vi "test_gpsparsing-dyy1.vi"() -> ()   [LabVIEW 2019]
panel:
  in  "rs232 input":string="INSPVAXA,USB3,0,51.0,FINESTEERING,2107,281115.600,02000000,471d,15824;INS_ALIGNMENT_COMPLETE,INS_RTKFIXED,37.37013888668,126.72084169564,9.8834,22.3000,0.0026,0.0071,0.0017,-0.044376618,-0.064379115,35.875304095,0.1980,0.1670,0.2645,0.0373,0.0373,0.0312,0.3280,0.3375,5.4270,0f000015,0*6411398e\n\t"
  in  "raw sentences":string="#INSPVAXA,USB1,0,48.5,FINESTEERING,2089,274774.000,02000000,471d,15824;INS_SOLUTION_GOOD,INS_PSRSP,37.29130387489,127.14837722879,180.1875,23.4000,-0.0013,0.0009,0.0006,0.551873578,0.409746986,245.238942969,0.9351,1.1352,1.8213,0.0013,0.0013,0.0011,0.5220,0.5327,0.0827,0f000044,0*ebcb680a\r\n#INSPVAXA,USB1,0,46.0,FINESTEERING,2089,274774.500,02000000,471d,15824;INS_SOLUTION_GOOD,INS_PSRSP,37.29130387510,127.14837722993,180.1872,23.4000,-0.0011,0.0012,0.0001,0.555094420,0.409664932,245.237706469,0.9353,1.1353,1.8214,0.0013,0.0013,0.0011,0.5219,0.5326,0.0825,0f000044,0*777011ab\r\n#INSPVAXA,USB1,0,43.5,FINESTEERING,2089,274833.000,02000000,471d,15824;INS_SOLUTION_GOOD,INS_PSRSP,37.29130384920,127.14837718901,180.1935,23.4000,0.0010,0.0016,0.0001,0.586508598,0.420271557,245.302228537,0.9484,1.1462,1.8280,0.0013,0.0013,0.0011,0.5170,0.5273,0.0804,0f000044,0*4ffbbfb3\r\n#INSPVAXA,USB1,0,43.5,FINESTEERING,2089,274833.500,02000000,471d,15824;INS_SOLUTION_GOOD,INS_PSRSP,37.29130384818,127.14837718608,180.1933,23.4000,0.0010,0.0008,-0.0005,0.588637214,0.418146390,245.299960128,0.9485,1.1462,1.8281,0.0013,0.0013,0.0011,0.5169,0.5272,0.0802,0f000044,0*aa66d913\r\n#INSPVAXA,USB1,0,45.5,FINESTEERING,2089,274834.000,02000000,471d,15824;INS_SOLUTION_GOOD,INS_PSRSP,37.29130384916,127.14837718345,180.1929,23.4000,0.0015,0.0004,-0.0005,0.590372743,0.418871037,245.299569777,0.9485,1.1462,1.8281,0.0013,0.0013,0.0011,0.5169,0.5272,0.0802,0f000044,0*83fcb3d7\r\n#INSPVAXA,USB1,0,41.5,FINESTEERING,2089,274834.500,02000000,471d,15824;INS_SOLUTION_GOOD,INS_PSRSP,37.29130384548,127.14837718346,180.1928,23.4000,0.0001,0.0000,-0.0006,0.589131920,0.420278401,245.300229975,0.9486,1.1463,1.8281,0.0013,0.0013,0.0011,0.5168,0.5272,0.0801,0f000044,0*a2231570\r\n#INSPVAXA,USB1,0,41.5,FINESTEERING,2089,274835.000,02000000,471d,15824;INS_SOLUTION_GOOD,INS_PSRSP,37.29130384335,127.14837718516,180.1928,23.4000,0.0007,0.0007,-0.0001,0.587725622,0.422163583,245.298857552,0.9486,1.1463,1.8281,0.0013,0.0013,0.0011,0.5168,0.5272,0.0801,0f000044,0*a4c2c19e\r\n#INSPVAXA,USB1,0,41.5,FINESTEERING,2089,274835.500,02000000,471d,15824;INS_SOLUTION_GOOD,INS_PSRSP,37.29130384579,127.14837718571,180.1931,23.4000,0.0007,0.0010,0.0003,0.585320450,0.422207630,245.298031526,0.9487,1.1464,1.8282,0.0013,0.0013,0.0011,0.5167,0.5271,0.0801,0f000044,0*54c9d66f\r\n#INSPVAXA,USB1,0,42.0,FINESTEERING,2089,274836.000,02000000,471d,15824;INS_SOLUTION_GOOD,INS_PSRSP,37.29130384541,127.14837718965,180.1938,23.4000,-0.0004,0.0017,0.0013,0.584834735,0.420652895,245.296961531,0.9487,1.1464,1.8282,0.0013,0.0013,0.0011,0.5167,0.5271,0.0801,0f000044,0*6e73d9be\r\n#INSPVAXA,USB1,0,42.0,FINESTEERING,2089,274836.500,02000000,471d,15824;INS_SOLUTION_GOOD,INS_PSRSP,37.29130384325,127.14837718988,180.1936,23.4000,-0.0007,0.0022,0.0002,0.586640561,0.420248412,245.293704375,0.9488,1.1465,1.8282,0.0013,0.0013,0.0011,0.5166,0.5269,0.0800,0f000044,0*6525d3dd\r\n#INSPVAXA,USB1,0,46.5,FINESTEERING,2089,274837.000,02000000,471d,15824;INS_SOLUTION_GOOD,INS_PSRSP,37.29130384316,127.14837719750,180.1935,23.4000,0.0006,0.0025,0.0009,0.587577449,0.421045753,245.294799323,0.9488,1.1465,1.8282,0.0013,0.0013,0.0011,0.5166,0.5269,0.0800,0f000044,0*355fafb1\r\n#INSPVAXA,USB1,0,45.0,FINESTEERING,2089,274837.500,02000000,471d,15824;INS_SOLUTION_GOOD,INS_PSRSP,37.29130384444,127.14837719525,180.1933,23.4000,0.0006,0.0018,0.0013,0.584921247,0.421902824,245.290603324,0.9489,1.1466,1.8283,0.0013,0.0013,0.0011,0.5165,0.5268,0.0788,0f000054,0*624cd272\r\n#INSPVAXA,USB1,0,45.0,FINESTEERING,2089,274838.000,02000000,471d,15824;INS_SOLUTION_GOOD,INS_PSRSP,37.29130384668,127.14837719935,180.1933,23.4000,0.0015,0.0021,0.0029,0.572458182,0.422818028,245.285259282,0.9489,1.1466,1.8283,0.0013,0.0013,0.0011,0.5165,0.5268,0.0788,0f000054,0*f0969d6b\r\n#INSPVAXA,USB1,0,45.0,FINESTEERING,2089,274838.500,02000000,471d,15824;INS_SOLUTION_GOOD,INS_PSRSP,37.29130385339,127.14837721565,180.1933,23.4000,0.0025,0.0026,0.0011,0.577250419,0.424806742,245.288423965,0.9494,1.1470,1.8285,0.0093,0.0093,0.0089,0.5166,0.5269,0.0786,0f000050,0*ea9babb5\r\n#INSPVAXA,USB1,0,47.5,FINESTEERING,2089,274839.000,02000000,471d,15824;INS_SOLUTION_GOOD,INS_PSRSP,37.29130386328,127.14837723993,180.1932,23.4000,0.0017,0.0052,-0.0009,0.582029495,0.425850241,245.288353682,0.9494,1.1470,1.8285,0.0093,0.0093,0.0089,0.5166,0.5269,0.0786,0f000050,0*7585d0cb\r\n#INSPVAXA,USB1,0,47.0,FINESTEERING,2089,274839.500,02000000,471d,15824;INS_SOLUTION_GOOD,INS_PSRSP,37.29130385792,127.14837721902,180.1939,23.4000,0.0020,0.0033,-0.0000,0.584809398,0.427483800,245.289111380,0.9494,1.1470,1.8285,0.0014,0.0014,0.0011,0.5164,0.5268,0.0774,0f000054,1*4ac2f79a\r\n#INSPVAXA,USB1,0,47.0,FINESTEERING,2089,274840.000,02000000,471d,15824;INS_SOLUTION_GOOD,INS_PSRSP,37.29130385001,127.14837719578,180.1947,23.4000,0.0002,0.0006,0.0013,0.582864364,0.430853297,245.289734886,0.9494,1.1470,1.8285,0.0014,0.0014,0.0011,0.5164,0.5268,0.0774,0f000054,1*ff928a43\r\n#INSPVAXA,USB1,0,45.5,FINESTEERING,2089,274840.500,02000000,471d,15824;INS_SOLUTION_GOOD,INS_PSRSP,37.29130384317,127.14837719277,180.1946,23.4000,-0.0003,0.0001,0.0018,0.589516020,0.432666121,245.285723932,0.9495,1.1471,1.8286,0.0013,0.0013,0.0011,0.5162,0.5266,0.0765,0f000054,0*c3e6f0a5\r\n#INSPVAXA,USB1,0,45.5,FINESTEERING,2089,274841.000,02000000,471d,15824;INS_SOLUTION_GOOD,INS_PSRSP,37.29130383148,127.14837719105,180.1944,23.4000,-0.0023,0.0009,0.0013,0.604493717,0.434742929,245.281282043,0.9495,1.1471,1.8286,0.0013,0.0013,0.0011,0.5162,0.5266,0.0765,0f000054,0*7f3014c1\r\n#INSPVAXA,USB1,0,45.0,FINESTEERING,2089,274841.500,02000000,471d,15824;INS_SOLUTION_GOOD,INS_PSRSP,37.29130383115,127.14837718814,180.1940,23.4000,-0.0016,-0.0003,0.0001,0.617397798,0.434325557,245.271090749,0.9496,1.1472,1.8287,0.0013,0.0013,0.0011,0.5161,0.5264,0.0756,0f000054,0*8095e45b\r\n#INSPVAXA,USB1,0,45.0,FINESTEERING,2089,274842.000,02000000,471d,15824;INS_SOLUTION_GOOD,INS_PSRSP,37.29130383593,127.14837718812,180.1938,23.4000,-0.0011,0.0010,0.0008,0.620982729,0.439593409,245.265361274,0.9496,1.1472,1.8287,0.0013,0.0013,0.0011,0.5161,0.5264,0.0756,0f000054,0*e9d9bf62\r\n#INSPVAXA,USB1,0,44.5,FINESTEERING,2089,274842.500,02000000,471d,15824;INS_SOLUTION_GOOD,INS_PSRSP,37.29130384482,127.14837719080,180.1937,23.4000,0.0016,0.0013,0.0009,0.605631119,0.442829775,245.265554584,0.9497,1.1473,1.8287,0.0013,0.0013,0.0011,0.5160,0.5262,0.0754,0f000044,0*5f93a9d6\r\n#INSPVAXA,USB1,0,44.5,FINESTEERING,2089,274843.000,02000000,471d,15824;INS_SOLUTION_GOOD,INS_PSRSP,37.29130385974,127.14837719761,180.1937,23.4000,0.0030,0.0017,0.0023,0.612022246,0.444081560,245.266194594,0.9497,1.1473,1.8287,0.0013,0.0013,0.0011,0.5160,0.5262,0.0754,0f000044,0*02985e66\r\n#INSPVAXA,USB1,0,44.0,FINESTEERING,2089,274843.500,02000000,471d,15824;INS_SOLUTION_GOOD,INS_PSRSP,37.29130385669,127.14837719988,180.1927,23.4000,0.0035,0.0029,-0.0003,0.612226712,0.441870822,245.266043101,0.9499,1.1474,1.8288,0.0013,0.0013,0.0011,0.5159,0.5261,0.0745,0f000054,0*83215f55\r\n#INSPVAXA,USB1,0,44.0,FINESTEERING,2089,274844.000,02000000,471d,15824;INS_SOLUTION_GOOD,INS_PSRSP,37.29130385766,127.14837720982,180.1916,23.4000,0.0039,0.0038,-0.0022,0.611461962,0.438198250,245.264691822,0.9499,1.1474,1.8288,0.0013,0.0013,0.0011,0.5159,0.5261,0.0745,0f000054,0*fb962826\r\n#INSPVAXA,USB1,0,43.0,FINESTEERING,2089,274844.500,02000000,471d,15824;INS_SOLUTION_GOOD,INS_PSRSP,37.29130385088,127.14837720148,180.1930,23.4000,0.0014,0.0032,-0.0007,0.622605176,0.439726412,245.265560703,0.9500,1.1475,1.8288,0.0013,0.0013,0.0011,0.5158,0.5260,0.0742,0f000044,0*d6a7df55\r\n#INSPVAXA,USB1,0,43.0,FINESTEERING,2089,274845.000,02000000,471d,15824;INS_SOLUTION_GOOD,INS_PSRSP,37.29130384875,127.14837719586,180.1943,23.4000,0.0017,0.0016,0.0007,0.629621138,0.435407053,245.265376008,0.9500,1.1475,1.8288,0.0013,0.0013,0.0011,0.5158,0.5260,0.0742,0f000044,0*9a02e1b8\r\n#INSPVAXA,USB1,0,43.0,FINESTEERING,2089,274845.500,02000000,471d,15824;INS_SOLUTION_GOOD,INS_PSRSP,37.29130384480,127.14837719107,180.1934,23.4000,0.0013,0.0014,-0.0020,0.625363002,0.431760314,245.263604467,0.9501,1.1476,1.8289,0.0013,0.0013,0.0011,0.5157,0.5258,0.0738,0f000054,0*007f2e1b\r\n#INSPVAXA,USB1,0,44.5,FINESTEERING,2089,274846.000,02000000,471d,15824;INS_SOLUTION_GOOD,INS_PSRSP,37.29130384319,127.14837718852,180.1923,23.4000,0.0017,0.0002,-0.0005,0.610919166,0.435153624,245.267483815,0.9501,1.1476,1.8289,0.0013,0.0013,0.0011,0.5157,0.5258,0.0738,0f000054,0*b5f3ee81\r\n#INSPVAXA,USB1,0,44.5,FINESTEERING,2089,274846.500,02000000,471d,15824;INS_SOLUTION_GOOD,INS_PSRSP,37.29130384630,127.14837718697,180.1925,23.4000,0.0021,-0.0006,-0.0005,0.638769476,0.428687028,245.270913494,0.9502,1.1477,1.8290,0.0013,0.0013,0.0011,0.5157,0.5257,0.0732,0f000054,0*5038ed49\r\n#INSPVAXA,USB1,0,45.5,FINESTEERING,2089,274847.000,02000000,471d,15824;INS_SOLUTION_GOOD,INS_PSRSP,37.29130385570,127.14837718789,180.1924,23.4000,0.0031,0.0004,-0.0013,0.595340822,0.432590705,245.280511440,0.9502,1.1477,1.8290,0.0013,0.0013,0.0011,0.5157,0.5257,0.0732,0f000054,0*63a9ce85\r\n#INSPVAXA,USB1,0,45.5,FINESTEERING,2089,274847.500,02000000,471d,15824;INS_SOLUTION_GOOD,INS_PSRSP,37.29130384697,127.14837718770,180.1930,23.4000,0.0027,0.0009,-0.0013,0.585915070,0.434608590,245.296052535,0.9503,1.1478,1.8290,0.0013,0.0013,0.0011,0.5156,0.5255,0.0727,0f000054,0*8727ca3a\r\n#INSPVAXA,USB1,0,47.0,FINESTEERING,2089,274848.000,02000000,471d,15824;INS_SOLUTION_GOOD,INS_PSRSP,37.29130384047,127.14837719167,180.1933,23.4000,-0.0007,0.0001,-0.0004,0.580727730,0.433378186,245.297804962,0.9503,1.1478,1.8290,0.0013,0.0013,0.0011,0.5156,0.5255,0.0727,0f000054,0*12b0bc20\r\n#INSPVAXA,USB1,0,47.0,FINESTEERING,2089,274848.500,02000000,471d,15824;INS_SOLUTION_GOOD,INS_PSRSP,37.29130384306,127.14837719348,180.1930,23.4000,0.0022,0.0007,-0.0006,0.580866513,0.432295299,245.319835018,0.9504,1.1479,1.8291,0.0013,0.0013,0.0011,0.5153,0.5254,0.0727,0f000054,0*ec30085f\r\n#INSPVAXA,USB1,0,47.0,FINESTEERING,2089,274849.000,02000000,471d,15824;INS_SOLUTION_GOOD,INS_PSRSP,37.29130384731,127.14837719041,180.1926,23.4000,0.0009,0.0008,-0.0020,0.585803127,0.428708561,245.313218235,0.9504,1.1479,1.8291,0.0013,0.0013,0.0011,0.5153,0.5254,0.0727,0f000054,0*28d56c23\r\n#INSPVAXA,USB1,0,46.5,FINESTEERING,2089,274849.500,02000000,471d,15824;INS_SOLUTION_GOOD,INS_PSRSP,37.29130384758,127.14837718974,180.1928,23.4000,0.0012,-0.0003,-0.0019,0.588947359,0.426740055,245.315643224,0.9505,1.1479,1.8291,0.0013,0.0013,0.0011,0.5152,0.5253,0.0727,0f000054,0*c2e00834\r\n#INSPVAXA,USB1,0,46.5,FINESTEERING,2089,274850.000,02000000,471d,15824;INS_SOLUTION_GOOD,INS_PSRSP,37.29130385122,127.14837718979,180.1929,23.4000,0.0015,-0.0010,-0.0009,0.581528107,0.426050857,245.323456815,0.9505,1.1479,1.8291,0.0013,0.0013,0.0011,0.5152,0.5253,0.0727,0f000054,0*1f70a6a8\r\n#INSPVAXA,USB1,0,46.5,FINESTEERING,2089,274850.500,02000000,471d,15824;INS_SOLUTION_GOOD,INS_PSRSP,37.29130385052,127.14837719501,180.1930,23.4000,0.0017,0.0018,-0.0007,0.585928565,0.430332055,245.313181688,0.9506,1.1480,1.8292,0.0013,0.0013,0.0011,0.5151,0.5251,0.0726,0f000154,0*17301aa5\r\n#INSPVAXA,USB1,0,49.0,FINESTEERING,2089,274851.000,02000000,471d,15824;INS_SOLUTION_GOOD,INS_PSRSP,37.29130385542,127.14837720662,180.1929,23.4000,0.0024,0.0025,-0.0015,0.585449635,0.431152918,245.300968505,0.9506,1.1480,1.8292,0.0013,0.0013,0.0011,0.5151,0.5251,0.0726,0f000154,0*03de2636\r\n#INSPVAXA,USB1,0,47.0,FINESTEERING,2089,274851.500,02000000,471d,15824;INS_SOLUTION_GOOD,INS_PSRSP,37.29130385416,127.14837719820,180.1933,23.4000,0.0028,0.0008,0.0003,0.574219615,0.429594104,245.299898769,0.9507,1.1481,1.8292,0.0013,0.0013,0.0011,0.5149,0.5250,0.0719,0f000154,0*b7f115ad\r\n#INSPVAXA,USB1,0,47.0,FINESTEERING,2089,274852.000,02000000,471d,15824;INS_SOLUTION_GOOD,INS_PSRSP,37.29130385933,127.14837719142,180.1936,23.4000,0.0034,0.0001,0.0002,0.602150238,0.421206875,245.297537653,0.9507,1.1481,1.8292,0.0013,0.0013,0.0011,0.5149,0.5250,0.0719,0f000154,0*adddd9a6\r\n#INSPVAXA,USB1,0,45.0,FINESTEERING,2089,274852.500,02000000,471d,15824;INS_SOLUTION_GOOD,INS_PSRSP,37.29130385641,127.14837719046,180.1925,23.4000,0.0036,0.0006,-0.0019,0.602525216,0.420748496,245.291164286,0.9508,1.1482,1.8293,0.0013,0.0013,0.0011,0.5149,0.5248,0.0712,0f000154,0*59076c56\r\n#INSPVAXA,USB1,0,45.0,FINESTEERING,2089,274853.000,02000000,471d,15824;INS_SOLUTION_GOOD,INS_PSRSP,37.29130385932,127.14837719010,180.1910,23.4000,0.0033,-0.0004,-0.0028,0.587257028,0.423997918,245.289640051,0.9508,1.1482,1.8293,0.0013,0.0013,0.0011,0.5149,0.5248,0.0712,0f000154,0*0778e67e\r\n#INSPVAXA,USB1,0,45.0,FINESTEERING,2089,274853.500,02000000,471d,15824;INS_SOLUTION_GOOD,INS_PSRSP,37.29130371848,127.14837706011,180.1620,23.4000,0.0027,0.0003,-0.0009,0.574716234,0.423962622,245.287552041,0.9348,1.1276,1.8079,0.0013,0.0013,0.0011,0.5148,0.5247,0.0706,0f000055,0*7912a674\r\n#INSPVAXA,USB1,0,50.5,FINESTEERING,2089,274854.000,02000000,471d,15824;INS_SOLUTION_GOOD,INS_PSRSP,37.29130357736,127.14837692724,180.1315,23.4000,0.0027,-0.0000,0.0010,0.593573985,0.422376393,245.286718200,0.9348,1.1276,1.8079,0.0013,0.0013,0.0011,0.5148,0.5247,0.0706,0f000055,0*0bc1c9d9\r\n#INSPVAXA,USB1,0,49.5,FINESTEERING,2089,274854.500,02000000,471d,15824;INS_SOLUTION_GOOD,INS_PSRSP,37.29130344177,127.14837679808,180.1007,23.4000,0.0027,0.0002,-0.0006,0.595349698,0.420604015,245.293380432,0.9316,1.1180,1.7938,0.0013,0.0013,0.0011,0.5146,0.5245,0.0699,0f000055,0*57c3e6fd\r\n#INSPVAXA,USB1,0,49.5,FINESTEERING,2089,274855.000,02000000,471d,15824;INS_SOLUTION_GOOD,INS_PSRSP,37.29130331141,127.14837666894,180.0693,23.4000,0.0035,0.0010,-0.0026,0.608069981,0.421964756,245.302966124,0.9316,1.1180,1.7938,0.0013,0.0013,0.0011,0.5146,0.5245,0.0699,0f000055,0*cc081c3a\r\n#INSPVAXA,USB1,0,49.5,FINESTEERING,2089,274855.500,02000000,471d,15824;INS_SOLUTION_GOOD,INS_PSRSP,37.29130318484,127.14837654183,180.0416,23.4000,0.0030,0.0004,-0.0030,0.598292360,0.422007791,245.320543433,0.9284,1.1089,1.7802,0.0013,0.0013,0.0011,0.5146,0.5244,0.0693,0f000055,0*07a8aa8c\r\n#INSPVAXA,USB1,0,49.5,FINESTEERING,2089,274856.000,02000000,471d,15824;INS_SOLUTION_GOOD,INS_PSRSP,37.29130306029,127.14837641048,180.0134,23.4000,0.0016,0.0007,-0.0021,0.585405768,0.419049251,245.328126079,0.9284,1.1089,1.7802,0.0013,0.0013,0.0011,0.5146,0.5244,0.0693,0f000055,0*b15bf8d5\r\n#INSPVAXA,USB1,0,46.5,FINESTEERING,2089,274856.500,02000000,471d,15824;INS_SOLUTION_GOOD,INS_PSRSP,37.29130294212,127.14837629270,179.9885,23.4000,0.0022,0.0002,-0.0011,0.611087802,0.415829090,245.327294205,0.9253,1.1003,1.7671,0.0013,0.0013,0.0011,0.5144,0.5243,0.0693,0f000055,0*d8695a29\r\n#INSPVAXA,USB1,0,46.5,FINESTEERING,2089,274857.000,02000000,471d,15824;INS_SOLUTION_GOOD,INS_PSRSP,37.29130282516,127.14837617164,179.9628,23.4000,0.0025,-0.0024,-0.0003,0.610710666,0.416879256,245.329332541,0.9253,1.1003,1.7671,0.0013,0.0013,0.0011,0.5144,0.5243,0.0693,0f000055,0*2df2750a\r\n#INSPVAXA,USB1,0,46.5,FINESTEERING,2089,274857.500,02000000,471d,15824;INS_SOLUTION_GOOD,INS_PSRSP,37.29130269900,127.14837605784,179.9379,23.4000,-0.0037,-0.0010,0.0004,0.604642941,0.414177968,245.327268875,0.9223,1.0920,1.7545,0.0013,0.0013,0.0011,0.5143,0.5242,0.0687,0f000055,0*5f2d8b68\r\n#INSPVAXA,USB1,0,50.0,FINESTEERING,2089,274858.000,02000000,471d,15824;INS_SOLUTION_GOOD,INS_PSRSP,37.29130256253,127.14837593545,179.9126,23.4000,-0.0034,-0.0026,0.0011,0.619142357,0.411036243,245.327897197,0.9223,1.0920,1.7545,0.0013,0.0013,0.0011,0.5143,0.5242,0.0687,0f000055,0*59bcebc3\r\n#INSPVAXA,USB1,0,46.5,FINESTEERING,2089,274858.500,02000000,471d,15824;INS_SOLUTION_GOOD,INS_PSRSP,37.29130246087,127.14837583393,179.8879,23.4000,-0.0040,-0.0040,0.0016,0.604247748,0.416532560,245.319150499,0.9193,1.0841,1.7424,0.0013,0.0013,0.0011,0.5141,0.5239,0.0681,0f000055,0*a00f20b9\r\n#INSPVAXA,USB1,0,46.5,FINESTEERING,2089,274859.000,02000000,471d,15824;INS_SOLUTION_GOOD,INS_PSRSP,37.29130235836,127.14837573357,179.8629,23.4000,-0.0017,0.0010,-0.0003,0.593891010,0.422439967,245.326322938,0.9193,1.0841,1.7424,0.0013,0.0013,0.0011,0.5141,0.5239,0.0681,0f000055,0*a300ea15\r\n#INSPVAXA,USB1,0,46.5,FINESTEERING,2089,274859.500,02000000,471d,15824;INS_SOLUTION_GOOD,INS_PSRSP,37.29130184663,127.14837554476,179.9303,23.4000,0.0020,-0.0004,-0.0004,0.604038265,0.423564477,245.322788284,0.9100,1.0764,1.7185,0.0013,0.0013,0.0011,0.5140,0.5237,0.0675,0f000055,0*5c1099b4\r\n#INSPVAXA,USB1,0,47.0,FINESTEERING,2089,274860.000,02000000,471d,15824;INS_SOLUTION_GOOD,INS_PSRSP,37.29130131283,127.14837535131,180.0020,23.4000,0.0014,0.0017,0.0010,0.598838351,0.427865857,245.324862562,0.9100,1.0764,1.7185,0.0013,0.0013,0.0011,0.5140,0.5237,0.0675,0f000055,0*fe87ed6a\r\n#INSPVAXA,USB1,0,45.5,FINESTEERING,2089,274860.500,02000000,471d,15824;INS_SOLUTION_GOOD,INS_PSRSP,37.29130073894,127.14837514216,180.0820,23.4000,-0.0006,-0.0001,0.0008,0.602063249,0.428393600,245.328127358,0.9010,1.0691,1.6952,0.0013,0.0013,0.0011,0.5139,0.5236,0.0668,0f000055,0*f96cb01e\r\n#INSPVAXA,USB1,0,45.5,FINESTEERING,2089,274861.000,02000000,471d,15824;INS_SOLUTION_GOOD,INS_PSRSP,37.29130015247,127.14837492678,180.1637,23.4000,-0.0008,-0.0007,0.0006,0.600535903,0.427391101,245.325502543,0.9010,1.0691,1.6952,0.0013,0.0013,0.0011,0.5139,0.5236,0.0668,0f000055,0*01e3a804\r\n#INSPVAXA,USB1,0,45.5,FINESTEERING,2089,274861.500,02000000,471d,15824;INS_SOLUTION_GOOD,INS_PSRSP,37.29129962771,127.14837473344,180.2380,23.4000,0.0007,-0.0000,-0.0002,0.605081346,0.428771957,245.324679101,0.8926,1.0622,1.6728,0.0013,0.0013,0.0011,0.5138,0.5235,0.0662,0f000055,0*7cf27d00\r\n#INSPVAXA,USB1,0,45.5,FINESTEERING,2089,274862.000,02000000,471d,15824;INS_SOLUTION_GOOD,INS_PSRSP,37.29129910049,127.14837453785,180.3130,23.4000,0.0012,0.0004,-0.0011,0.606547987,0.427565132,245.323707444,0.8926,1.0622,1.6728,0.0013,0.0013,0.0011,0.5138,0.5235,0.0662,0f000055,0*a053525a\r\n#INSPVAXA,USB1,0,45.5,FINESTEERING,2089,274862.500,02000000,471d,15824;INS_SOLUTION_GOOD,INS_PSRSP,37.29129862218,127.14837437155,180.3848,23.4000,0.0012,-0.0012,0.0017,0.609120994,0.423744316,245.328206368,0.8844,1.0556,1.6510,0.0012,0.0012,0.0011,0.5137,0.5235,0.0655,0f000055,0*a456a61a\r\n#INSPVAXA,USB1,0,46.5,FINESTEERING,2089,274863.000,02000000,471d,15824;INS_SOLUTION_GOOD,INS_PSRSP,37.29129813853,127.14837420331,180.4578,23.4000,0.0010,-0.0005,0.0010,0.602661252,0.422338127,245.331968822,0.8844,1.0556,1.6510,0.0012,0.0012,0.0011,0.5137,0.5235,0.0655,0f000055,0*1554e39a\r\n#INSPVAXA,USB1,0,46.5,FINESTEERING,2089,274863.500,02000000,471d,15824;INS_SOLUTION_GOOD,INS_PSRSP,37.29129811823,127.14837413488,180.4341,23.4000,0.0002,-0.0005,0.0007,0.602768734,0.421866591,245.330987402,0.8829,1.0494,1.6419,0.0012,0.0012,0.0011,0.5136,0.5233,0.0649,0f000055,0*ea05af05\r\n#INSPVAXA,USB1,0,47.0,FINESTEERING,2089,274864.000,02000000,471d,15824;INS_SOLUTION_GOOD,INS_PSRSP,37.29129811114,127.14837406741,180.4071,23.4000,-0.0003,-0.0008,0.0012,0.594006086,0.419586959,245.329450491,0.8829,1.0494,1.6419,0.0012,0.0012,0.0011,0.5136,0.5233,0.0649,0f000055,0*39da8561\r\n#INSPVAXA,USB1,0,46.0,FINESTEERING,2089,274864.500,02000000,471d,15824;INS_SOLUTION_GOOD,INS_PSRSP,37.29129763515,127.14837392008,180.4809,23.4000,0.0009,-0.0003,0.0015,0.591614221,0.421635032,245.331904041,0.8747,1.0433,1.6208,0.0012,0.0012,0.0011,0.5135,0.5232,0.0642,0f000055,0*abb8aca2\r\n#INSPVAXA,USB1,0,46.0,FINESTEERING,2089,274865.000,02000000,471d,15824;INS_SOLUTION_GOOD,INS_PSRSP,37.29129713783,127.14837376713,180.5596,23.4000,0.0006,0.0006,0.0014,0.594757188,0.424159678,245.334157179,0.8747,1.0433,1.6208,0.0012,0.0012,0.0011,0.5135,0.5232,0.0642,0f000055,0*fc500cf6\r\n#INSPVAXA,USB1,0,46.0,FINESTEERING,2089,274865.500,02000000,471d,15824;INS_SOLUTION_GOOD,INS_PSRSP,37.29129664620,127.14837358797,180.6297,23.4000,0.0018,-0.0014,0.0013,0.595020918,0.424389592,245.336049519,0.8664,1.0371,1.5997,0.0012,0.0012,0.0011,0.5134,0.5231,0.0635,0f000055,0*b8b974b9\r\n#INSPVAXA,USB1,0,46.0,FINESTEERING,2089,274866.000,02000000,471d,15824;INS_SOLUTION_GOOD,INS_PSRSP,37.29129615440,127.14837340087,180.7009,23.4000,0.0053,-0.0020,0.0023,0.595443162,0.426827875,245.337186891,0.8664,1.0371,1.5997,0.0012,0.0012,0.0011,0.5134,0.5231,0.0635,0f000055,0*f5d76d32\r\n#INSPVAXA,USB1,0,46.0,FINESTEERING,2089,274866.500,02000000,471d,15824;INS_SOLUTION_GOOD,INS_PSRSP,37.29129616080,127.14837337991,180.7039,23.4000,0.0061,-0.0022,0.0013,0.594683328,0.427337075,245.340623936,0.8792,1.0477,1.6066,0.0075,0.0075,0.0073,0.5134,0.5231,0.0634,0f000150,0*bfe5e378\r\n#INSPVAXA,USB1,0,49.0,FINESTEERING,2089,274867.000,02000000,471d,15824;INS_SOLUTION_GOOD,INS_PSRSP,37.29129619014,127.14837336349,180.7047,23.4000,0.0071,-0.0031,0.0021,0.588073762,0.429417131,245.343896479,0.8792,1.0477,1.6066,0.0075,0.0075,0.0073,0.5134,0.5231,0.0634,0f000150,0*a3f56346\r\n#INSPVAXA,USB1,0,47.5,FINESTEERING,2089,274867.500,02000000,471d,15824;INS_SOLUTION_GOOD,INS_PSRSP,37.29129616233,127.14837338717,180.7042,23.4000,0.0057,-0.0006,0.0017,0.586248294,0.426049636,245.345160781,0.8793,1.0478,1.6067,0.0013,0.0013,0.0011,0.5132,0.5229,0.0629,0f000054,0*016d9dd1\r\n#INSPVAXA,USB1,0,47.5,FINESTEERING,2089,274868.000,02000000,471d,15824;INS_SOLUTION_GOOD,INS_PSRSP,37.29129613969,127.14837341229,180.7038,23.4000,0.0038,0.0002,0.0014,0.608576318,0.424144727,245.346624835,0.8793,1.0478,1.6067,0.0013,0.0013,0.0011,0.5132,0.5229,0.0629,0f000054,0*aa41e723\r\n#INSPVAXA,USB1,0,47.5,FINESTEERING,2089,274868.500,02000000,471d,15824;INS_SOLUTION_GOOD,INS_PSRSP,37.29129613379,127.14837340967,180.7035,23.4000,0.0031,-0.0022,0.0018,0.598614775,0.424399326,245.350390223,0.8794,1.0480,1.6068,0.0013,0.0013,0.0011,0.5131,0.5228,0.0626,0f000054,0*13e64130\r\n#INSPVAXA,USB1,0,49.0,FINESTEERING,2089,274869.000,02000000,471d,15824;INS_SOLUTION_GOOD,INS_PSRSP,37.29129613206,127.14837340426,180.7036,23.4000,0.0022,-0.0007,0.0016,0.603875615,0.425000213,245.357059747,0.8794,1.0480,1.6068,0.0013,0.0013,0.0011,0.5131,0.5228,0.0626,0f000054,0*e911c346\r\n#INSPVAXA,USB1,0,46.0,FINESTEERING,2089,274869.500,02000000,471d,15824;INS_SOLUTION_GOOD,INS_PSRSP,37.29129612727,127.14837340436,180.7035,23.4000,0.0037,0.0000,0.0018,0.593217302,0.423190884,245.353915706,0.8796,1.0481,1.6069,0.0013,0.0013,0.0011,0.5129,0.5226,0.0623,0f000054,0*1af8cbc1\r\n#INSPVAXA,USB1,0,46.0,FINESTEERING,2089,274870.000,02000000,471d,15824;INS_SOLUTION_GOOD,INS_PSRSP,37.29129612823,127.14837341106,180.7036,23.4000,0.0033,-0.0029,0.0013,0.588053000,0.426256122,245.364328613,0.8796,1.0481,1.6069,0.0013,0.0013,0.0011,0.5129,0.5226,0.0623,0f000054,0*393947a2\r\n#INSPVAXA,USB1,0,46.0,FINESTEERING,2089,274870.500,02000000,471d,15824;INS_SOLUTION_GOOD,INS_PSRSP,37.29129611988,127.14837342124,180.7036,23.4000,-0.0005,-0.0002,0.0015,0.579181444,0.421718816,245.356678428,0.8798,1.0482,1.6069,0.0013,0.0013,0.0011,0.5128,0.5225,0.0619,0f000054,0*9f61ccf9\r\n#INSPVAXA,USB1,0,46.5,FINESTEERING,2089,274871.000,02000000,471d,15824;INS_SOLUTION_GOOD,INS_PSRSP,37.29129610715,127.14837344092,180.7039,23.4000,0.0003,0.0022,0.0019,0.574163307,0.418359893,245.359211630,0.8798,1.0482,1.6069,0.0013,0.0013,0.0011,0.5128,0.5225,0.0619,0f000054,0*13af1866\r\n#INSPVAXA,USB1,0,46.5,FINESTEERING,2089,274871.500,02000000,471d,15824;INS_SOLUTION_GOOD,INS_PSRSP,37.29129610388,127.14837343476,180.7033,23.4000,-0.0031,0.0036,0.0006,0.562256928,0.420298473,245.361016185,0.8799,1.0484,1.6070,0.0013,0.0013,0.0011,0.5127,0.5224,0.0616,0f000054,0*6a34a145\r\n#INSPVAXA,USB1,0,47.5,FINESTEERING,2089,274872.000,02000000,471d,15824;INS_SOLUTION_GOOD,INS_PSRSP,37.29129609867,127.14837343167,180.7028,23.4000,-0.0040,0.0028,0.0003,0.555172991,0.420159860,245.362404089,0.8799,1.0484,1.6070,0.0013,0.0013,0.0011,0.5127,0.5224,0.0616,0f000054,0*7922a92c\r\n#INSPVAXA,USB1,0,47.5,FINESTEERING,2089,274872.500,02000000,471d,15824;INS_SOLUTION_GOOD,INS_PSRSP,37.29129610659,127.14837342345,180.7028,23.4000,-0.0029,0.0019,0.0000,0.553744177,0.422219874,245.361424871,0.8800,1.0485,1.6071,0.0013,0.0013,0.0011,0.5126,0.5223,0.0612,0f000054,0*5eadefc2\r\n#INSPVAXA,USB1,0,48.0,FINESTEERING,2089,274873.000,02000000,471d,15824;INS_SOLUTION_GOOD,INS_PSRSP,37.29129611274,127.14837341737,180.7029,23.4000,-0.0010,0.0014,0.0004,0.553262464,0.425519071,245.359892143,0.8800,1.0485,1.6071,0.0013,0.0013,0.0011,0.5126,0.5223,0.0612,0f000054,0*1dd6b914\r\n#INSPVAXA,USB1,0,47.0,FINESTEERING,2089,274873.500,02000000,471d,15824;INS_SOLUTION_GOOD,INS_PSRSP,37.29129611880,127.14837341572,180.7033,23.4000,-0.0000,0.0013,0.0005,0.549043260,0.425180742,245.358245933,0.8801,1.0486,1.6072,0.0013,0.0013,0.0011,0.5125,0.5221,0.0610,0f000054,0*30c4da77\r\n#INSPVAXA,USB1,0,47.0,FINESTEERING,2089,274874.000,02000000,471d,15824;INS_SOLUTION_GOOD,INS_PSRSP,37.29129612663,127.14837341599,180.7040,23.4000,0.0008,0.0012,0.0010,0.550522350,0.425290692,245.360780746,0.8801,1.0486,1.6072,0.0013,0.0013,0.0011,0.5125,0.5221,0.0610,0f000054,0*c4c8a5bb\r\n#INSPVAXA,USB1,0,46.0,FINESTEERING,2089,274874.500,02000000,471d,15824;INS_SOLUTION_GOOD,INS_PSRSP,37.29129612828,127.14837341546,180.7036,23.4000,0.0010,0.0011,0.0007,0.546173654,0.424177625,245.360098161,0.8803,1.0487,1.6072,0.0013,0.0013,0.0011,0.5124,0.5219,0.0607,0f000054,0*f301eded\r\n#INSPVAXA,USB1,0,46.0,FINESTEERING,2089,274875.000,02000000,471d,15824;INS_SOLUTION_GOOD,INS_PSRSP,37.29129612973,127.14837341576,180.7033,23.4000,0.0013,0.0009,0.0000,0.541215734,0.424206582,245.359664152,0.8803,1.0487,1.6072,0.0013,0.0013,0.0011,0.5124,0.5219,0.0607,0f000054,0*a00e3872\r\n#INSPVAXA,USB1,0,46.0,FINESTEERING,2089,274875.500,02000000,471d,15824;INS_SOLUTION_GOOD,INS_PSRSP,37.29129612475,127.14837341053,180.7028,23.4000,0.0002,-0.0003,-0.0004,0.547002338,0.421082053,245.361569216,0.8804,1.0488,1.6073,0.0013,0.0013,0.0011,0.5123,0.5217,0.0605,0f000054,0*8230e999\r\n#INSPVAXA,USB1,0,46.5,FINESTEERING,2089,274876.000,02000000,471d,15824;INS_SOLUTION_GOOD,INS_PSRSP,37.29129612106,127.14837340321,180.7023,23.4000,0.0002,-0.0006,-0.0012,0.551608602,0.419501813,245.361051793,0.8804,1.0488,1.6073,0.0013,0.0013,0.0011,0.5123,0.5217,0.0605,0f000054,0*cf65371f\r\n#INSPVAXA,USB1,0,46.5,FINESTEERING,2089,274876.500,02000000,471d,15824;INS_SOLUTION_GOOD,INS_PSRSP,37.29129612208,127.14837340675,180.7027,23.4000,0.0006,-0.0004,0.0000,0.549307254,0.420467396,245.361701249,0.8805,1.0489,1.6074,0.0012,0.0012,0.0011,0.5122,0.5215,0.0602,0f000054,0*8132308f\r\n#INSPVAXA,USB1,0,47.0,FINESTEERING,2089,274877.000,02000000,471d,15824;INS_SOLUTION_GOOD,INS_PSRSP,37.29129612899,127.14837341234,180.7033,23.4000,0.0021,0.0005,0.0006,0.550725794,0.419116319,245.357961941,0.8805,1.0489,1.6074,0.0012,0.0012,0.0011,0.5122,0.5215,0.0602,0f000054,0*6643ccab\r\n#INSPVAXA,USB1,0,47.0,FINESTEERING,2089,274877.500,02000000,471d,15824;INS_SOLUTION_GOOD,INS_PSRSP,37.29129612865,127.14837341039,180.7029,23.4000,0.0018,0.0002,-0.0005,0.551321835,0.418270107,245.358718362,0.8806,1.0490,1.6074,0.0012,0.0012,0.0011,0.5121,0.5212,0.0599,0f000054,0*5ee3f1a7\r\n#INSPVAXA,USB1,0,47.5,FINESTEERING,2089,274878.000,02000000,471d,15824;INS_SOLUTION_GOOD,INS_PSRSP,37.29129612878,127.14837341054,180.7023,23.4000,0.0004,0.0001,-0.0005,0.546964972,0.421152027,245.357711511,0.8806,1.0490,1.6074,0.0012,0.0012,0.0011,0.5121,0.5212,0.0599,0f000054,0*a3184f1a\r\n#INSPVAXA,USB1,0,47.5,FINESTEERING,2089,274878.500,02000000,471d,15824;INS_SOLUTION_GOOD,INS_PSRSP,37.29129612476,127.14837340984,180.7029,23.4000,-0.0005,-0.0004,0.0003,0.554489349,0.423948145,245.359502899,0.8808,1.0491,1.6075,0.0012,0.0012,0.0011,0.5120,0.5211,0.0596,0f000054,0*44dc7e35\r\n#INSPVAXA,USB1,0,48.5,FINESTEERING,2089,274879.000,02000000,471d,15824;INS_SOLUTION_GOOD,INS_PSRSP,37.29129611841,127.14837340676,180.7036,23.4000,-0.0007,-0.0007,0.0010,0.554733066,0.425455678,245.361084552,0.8808,1.0491,1.6075,0.0012,0.0012,0.0011,0.5120,0.5211,0.0596,0f000054,0*50da89eb\r\n#INSPVAXA,USB1,0,47.5,FINESTEERING,2089,274879.500,02000000,471d,15824;INS_SOLUTION_GOOD,INS_PSRSP,37.29129612066,127.14837340995,180.7032,23.4000,-0.0007,0.0001,0.0001,0.558276036,0.424708200,245.356775460,0.8809,1.0492,1.6076,0.0013,0.0013,0.0011,0.5119,0.5210,0.0601,0f000054,0*73780a10\r\n#INSPVAXA,USB1,0,47.5,FINESTEERING,2089,274880.000,02000000,471d,15824;INS_SOLUTION_GOOD,INS_PSRSP,37.29129612514,127.14837341450,180.7028,23.4000,0.0004,0.0011,-0.0005,0.571475369,0.429912271,245.353982735,0.8809,1.0492,1.6076,0.0013,0.0013,0.0011,0.5119,0.5210,0.0601,0f000054,0*d37bb229\r\n#INSPVAXA,USB1,0,46.5,FINESTEERING,2089,274880.500,02000000,471d,15824;INS_SOLUTION_GOOD,INS_PSRSP,37.29129612411,127.14837341605,180.7023,23.4000,0.0007,0.0017,-0.0012,0.569882680,0.430918054,245.353367154,0.8810,1.0493,1.6076,0.0013,0.0013,0.0011,0.5118,0.5209,0.0606,0f000054,0*a49baae6\r\n#INSPVAXA,USB1,0,46.5,FINESTEERING,2089,274881.000,02000000,471d,15824;INS_SOLUTION_GOOD,INS_PSRSP,37.29129612177,127.14837342345,180.7014,23.4000,-0.0007,0.0026,-0.0021,0.571097118,0.432128183,245.352632793,0.8810,1.0493,1.6076,0.0013,0.0013,0.0011,0.5118,0.5209,0.0606,0f000054,0*c497c499\r\n#INSPVAXA,USB1,0,46.5,FINESTEERING,2089,274881.500,02000000,471d,15824;INS_SOLUTION_GOOD,INS_PSRSP,37.29129612006,127.14837341653,180.7016,23.4000,-0.0010,0.0008,-0.0019,0.568056178,0.434224922,245.351229134,0.8811,1.0494,1.6077,0.0013,0.0013,0.0011,0.5118,0.5208,0.0609,0f000054,0*b9e9f07f\r\n#INSPVAXA,USB1,0,48.5,FINESTEERING,2089,274882.000,02000000,471d,15824;INS_SOLUTION_GOOD,INS_PSRSP,37.29129611784,127.14837340973,180.7016,23.4000,-0.0005,0.0008,-0.0017,0.569306107,0.434794439,245.348506056,0.8811,1.0494,1.6077,0.0013,0.0013,0.0011,0.5118,0.5208,0.0609,0f000054,0*d0e80636\r\n#INSPVAXA,USB1,0,48.0,FINESTEERING,2089,274882.500,02000000,471d,15824;INS_SOLUTION_GOOD,INS_PSRSP,37.29129612211,127.14837341172,180.7019,23.4000,0.0008,0.0013,-0.0017,0.567951973,0.438040408,245.347333063,0.8813,1.0495,1.6078,0.0013,0.0013,0.0011,0.5117,0.5208,0.0612,0f000054,0*8ceecd46\r\n#INSPVAXA,USB1,0,48.0,FINESTEERING,2089,274883.000,02000000,471d,15824;INS_SOLUTION_GOOD,INS_PSRSP,37.29129613288,127.14837342157,180.7019,23.4000,0.0032,0.0022,-0.0010,0.571684562,0.440407327,245.341991998,0.8813,1.0495,1.6078,0.0013,0.0013,0.0011,0.5117,0.5208,0.0612,0f000054,0*fb211987\r\n#INSPVAXA,USB1,0,46.0,FINESTEERING,2089,274883.500,02000000,471d,15824;INS_SOLUTION_GOOD,INS_PSRSP,37.29129613138,127.14837341951,180.7016,23.4000,0.0026,0.0022,-0.0020,0.566282828,0.436444176,245.336105943,0.8814,1.0496,1.6078,0.0013,0.0013,0.0011,0.5116,0.5207,0.0619,0f000054,0*4d1865ec\r\n#INSPVAXA,USB1,0,46.0,FINESTEERING,2089,274884.000,02000000,471d,15824;INS_SOLUTION_GOOD,INS_PSRSP,37.29129613231,127.14837342433,180.7012,23.4000,0.0013,0.0028,-0.0015,0.556862701,0.436683451,245.336796635,0.8814,1.0496,1.6078,0.0013,0.0013,0.0011,0.5116,0.5207,0.0619,0f000054,0*62aff0a1\r\n#INSPVAXA,USB1,0,46.0,FINESTEERING,2089,274884.500,02000000,471d,15824;INS_SOLUTION_GOOD,INS_PSRSP,37.29129613072,127.14837341898,180.7024,23.4000,0.0016,0.0019,0.0000,0.544667881,0.435253494,245.339787866,0.8815,1.0497,1.6079,0.0014,0.0014,0.0011,0.5115,0.5206,0.0625,0f000054,0*c991ff2a\r\n#INSPVAXA,USB1,0,48.5,FINESTEERING,2089,274885.000,02000000,471d,15824;INS_SOLUTION_GOOD,INS_PSRSP,37.29129613248,127.14837341613,180.7036,23.4000,0.0022,0.0017,0.0004,0.554979547,0.432786747,245.345114608,0.8815,1.0497,1.6079,0.0014,0.0014,0.0011,0.5115,0.5206,0.0625,0f000054,0*70c9fc55\r\n#INSPVAXA,USB1,0,47.5,FINESTEERING,2089,274885.500,02000000,471d,15824;INS_SOLUTION_GOOD,INS_PSRSP,37.29129613007,127.14837341623,180.7029,23.4000,0.0017,0.0012,-0.0012,0.554603932,0.429435956,245.351702366,0.8817,1.0498,1.6080,0.0014,0.0014,0.0011,0.5113,0.5204,0.0637,0f000054,0*8ff68242\r\n#INSPVAXA,USB1,0,47.5,FINESTEERING,2089,274886.000,02000000,471d,15824;INS_SOLUTION_GOOD,INS_PSRSP,37.29129613048,127.14837342172,180.7019,23.4000,0.0004,0.0021,-0.0015,0.549995061,0.428862607,245.359349814,0.8817,1.0498,1.6080,0.0014,0.0014,0.0011,0.5113,0.5204,0.0637,0f000054,0*4e0949e1\r\n#INSPVAXA,USB1,0,47.5,FINESTEERING,2089,274886.500,02000000,471d,15824;INS_SOLUTION_GOOD,INS_PSRSP,37.29129612734,127.14837342232,180.7020,23.4000,0.0000,0.0029,-0.0011,0.550255787,0.429595285,245.356182651,0.8818,1.0499,1.6081,0.0014,0.0014,0.0011,0.5113,0.5203,0.0651,0f000054,0*2ee9850d\r\n#INSPVAXA,USB1,0,48.5,FINESTEERING,2089,274887.000,02000000,471d,15824;INS_SOLUTION_GOOD,INS_PSRSP,37.29129612208,127.14837342788,180.7021,23.4000,-0.0005,0.0022,-0.0012,0.551821016,0.428591636,245.350229682,0.8818,1.0499,1.6081,0.0014,0.0014,0.0011,0.5113,0.5203,0.0651,0f000054,0*4d0c63d0\r\n#INSPVAXA,USB1,0,48.0,FINESTEERING,2089,274887.500,02000000,471d,15824;INS_SOLUTION_GOOD,INS_PSRSP,37.29129612160,127.14837342161,180.7022,23.4000,-0.0004,0.0017,-0.0012,0.550566085,0.429118165,245.350803996,0.8819,1.0501,1.6081,0.0014,0.0014,0.0011,0.5112,0.5203,0.0662,0f000054,0*a329d0f1\r\n#INSPVAXA,USB1,0,48.0,FINESTEERING,2089,274888.000,02000000,471d,15824;INS_SOLUTION_GOOD,INS_PSRSP,37.29129611996,127.14837341625,180.7022,23.4000,-0.0012,0.0008,-0.0012,0.550315057,0.427869625,245.349168441,0.8819,1.0501,1.6081,0.0014,0.0014,0.0011,0.5112,0.5203,0.0662,0f000054,0*e28460a8\r\n#INSPVAXA,USB1,0,47.0,FINESTEERING,2089,274888.500,02000000,471d,15824;INS_SOLUTION_GOOD,INS_PSRSP,37.29129612135,127.14837341466,180.7026,23.4000,-0.0008,0.0008,-0.0008,0.553204065,0.427354894,245.348475857,0.8820,1.0502,1.6082,0.0014,0.0014,0.0011,0.5111,0.5202,0.0670,0f000054,0*0b7a7f6d\r\n#INSPVAXA,USB1,0,47.0,FINESTEERING,2089,274889.000,02000000,471d,15824;INS_SOLUTION_GOOD,INS_PSRSP,37.29129612299,127.14837341846,180.7029,23.4000,0.0001,0.0020,-0.0001,0.552110930,0.427215097,245.342369198,0.8820,1.0502,1.6082,0.0014,0.0014,0.0011,0.5111,0.5202,0.0670,0f000054,0*d753ab21\r\n#INSPVAXA,USB1,0,47.0,FINESTEERING,2089,274889.500,02000000,471d,15824;INS_SOLUTION_GOOD,INS_PSRSP,37.29129612512,127.14837341890,180.7028,23.4000,-0.0000,0.0023,-0.0004,0.551179661,0.425073922,245.337435752,0.8822,1.0503,1.6083,0.0014,0.0014,0.0011,0.5110,0.5201,0.0675,0f000054,0*5c0e678b\r\n#INSPVAXA,USB1,0,48.0,FINESTEERING,2089,274890.000,02000000,471d,15824;INS_SOLUTION_GOOD,INS_PSRSP,37.29129612491,127.14837342285,180.7026,23.4000,-0.0007,0.0017,-0.0005,0.552467978,0.423041291,245.334974940,0.8822,1.0503,1.6083,0.0014,0.0014,0.0011,0.5110,0.5201,0.0675,0f000054,0*71c69c40\r\n#INSPVAXA,USB1,0,47.5,FINESTEERING,2089,274890.500,02000000,471d,15824;INS_SOLUTION_GOOD,INS_PSRSP,37.29129611839,127.14837342130,180.7032,23.4000,-0.0016,0.0024,0.0008,0.545912378,0.421928906,245.335647028,0.8823,1.0504,1.6083,0.0014,0.0014,0.0011,0.5109,0.5200,0.0678,0f000054,0*c60f5f17\r\n#INSPVAXA,USB1,0,47.5,FINESTEERING,2089,274891.000,02000000,471d,15824;INS_SOLUTION_GOOD,INS_PSRSP,37.29129610596,127.14837342803,180.7038,23.4000,-0.0032,0.0031,0.0011,0.551904024,0.419044569,245.334594576,0.8823,1.0504,1.6083,0.0014,0.0014,0.0011,0.5109,0.5200,0.0678,0f000054,0*ba1a294d\r\n#INSPVAXA,USB1,0,45.0,FINESTEERING,2089,274891.500,02000000,471d,15824;INS_SOLUTION_GOOD,INS_PSRSP,37.29129611095,127.14837342336,180.7032,23.4000,-0.0024,0.0026,0.0004,0.551707286,0.417318514,245.337325388,0.8824,1.0505,1.6084,0.0014,0.0014,0.0011,0.5107,0.5198,0.0680,0f000054,0*cd5b2ff4\r\n#INSPVAXA,USB1,0,45.0,FINESTEERING,2089,274892.000,02000000,471d,15824;INS_SOLUTION_GOOD,INS_PSRSP,37.29129611564,127.14837342273,180.7023,23.4000,-0.0005,0.0020,-0.0015,0.554665687,0.414561565,245.334115019,0.8824,1.0505,1.6084,0.0014,0.0014,0.0011,0.5107,0.5198,0.0680,0f000054,0*591179f7\r\n[USB1]#INSPVAXA,USB1,0,45.0,FINESTEERING,2089,274892.500,02000000,471d,15824;INS_SOLUTION_GOOD,INS_PSRSP,37.29129611903,127.14837341937,180.7023,23.4000,-0.0000,0.0020,-0.0022,0.553706522,0.412923899,245.332131853,0.8825,1.0506,1.6085,0.0013,0.0013,0.0011,0.5107,0.5198,0.0681,0f000054,0*af0d84eb\r\n#INSPVAXA,USB1,0,47.0,FINESTEERING,2089,274893.000,02000000,471d,15824;INS_SOLUTION_GOOD,INS_PSRSP,37.29129612276,127.14837341588,180.7019,23.4000,0.0010,0.0006,-0.0015,0.552759747,0.410805724,245.334223961,0.8825,1.0506,1.6085,0.0013,0.0013,0.0011,0.5107,0.5198,0.0681,0f000054,0*10f6e84c\r\n#INSPVAXA,USB1,0,46.0,FINESTEERING,2089,274893.500,02000000,471d,15824;INS_SOLUTION_GOOD,INS_PSRSP,37.29129612291,127.14837341052,180.7011,23.4000,-0.0000,-0.0011,-0.0032,0.547656129,0.409605873,245.339163651,0.8827,1.0507,1.6085,0.0013,0.0013,0.0011,0.5107,0.5197,0.0680,0f000054,0*dca6285e\r\n#INSPVAXA,USB1,0,46.0,FINESTEERING,2089,274894.000,02000000,471d,15824;INS_SOLUTION_GOOD,INS_PSRSP,37.29129612181,127.14837340219,180.6998,23.4000,0.0015,-0.0021,-0.0042,0.538172827,0.411040289,245.341117220,0.8827,1.0507,1.6085,0.0013,0.0013,0.0011,0.5107,0.5197,0.0680,0f000054,0*98b183d0\r\n#INSPVAXA,USB1,0,38.0,FINESTEERING,2089,274894.500,02000000,471d,15824;INS_SOLUTION_GOOD,INS_PSRSP,37.29129611253,127.14837340929,180.6998,23.4000,-0.0018,-0.0001,-0.0039,0.545272190,0.408193392,245.337409150,0.8828,1.0508,1.6086,0.0013,0.0013,0.0011,0.5105,0.5196,0.0678,0f000054,0*dcc810dc\r\n#INSPVAXA,USB1,0,38.0,FINESTEERING,2089,274895.000,02000000,471d,15824;INS_SOLUTION_GOOD,INS_PSRSP,37.29129610125,127.14837341717,180.6993,23.4000,-0.0027,0.0003,-0.0047,0.534134970,0.409161018,245.329507927,0.8828,1.0508,1.6086,0.0013,0.0013,0.0011,0.5105,0.5196,0.0678,0f000054,0*055d78d9\r\n#INSPVAXA,USB1,0,38.0,FINESTEERING,2089,274895.500,02000000,471d,15824;INS_SOLUTION_GOOD,INS_PSRSP,37.29129568163,127.14837350242,180.7741,23.4000,-0.0019,0.0015,-0.0041,0.549592840,0.410886710,245.331668254,0.8608,1.0335,1.5789,0.0013,0.0013,0.0011,0.5104,0.5196,0.0676,0f000055,0*6c994e54\r\n#INSPVAXA,USB1,0,47.0,FINESTEERING,2089,274896.000,02000000,471d,15824;INS_SOLUTION_GOOD,INS_PSRSP,37.29129523801,127.14837359721,180.8522,23.4000,-0.0016,0.0025,-0.0039,0.545156086,0.414753707,245.335191821,0.8608,1.0335,1.5789,0.0013,0.0013,0.0011,0.5104,0.5196,0.0676,0f000055,0*0522a3a2\r\n#INSPVAXA,USB1,0,47.0,FINESTEERING,2089,274896.500,02000000,471d,15824;INS_SOLUTION_GOOD,INS_PSRSP,37.29129483484,127.14837367907,180.9237,23.4000,-0.0003,0.0016,-0.0011,0.563215660,0.409887714,245.336369759,0.8506,1.0257,1.5564,0.0013,0.0013,0.0011,0.5103,0.5195,0.0673,0f000055,0*b9118182\r\n#INSPVAXA,USB1,0,50.5,FINESTEERING,2089,274897.000,02000000,471d,15824;INS_SOLUTION_GOOD,INS_PSRSP,37.29129442135,127.14837377007,180.9957,23.4000,-0.0016,0.0034,-0.0017,0.561308925,0.406998640,245.341534232,0.8506,1.0257,1.5564,0.0013,0.0013,0.0011,0.5103,0.5195,0.0673,0f000055,0*0e3ab7e7\r\n#INSPVAXA,USB1,0,48.5,FINESTEERING,2089,274897.500,02000000,471d,15824;INS_SOLUTION_GOOD,INS_PSRSP,37.29129405097,127.14837385413,181.0604,23.4000,-0.0018,0.0040,-0.0023,0.566207324,0.403915691,245.328055729,0.8411,1.0183,1.5353,0.0013,0.0013,0.0011,0.5102,0.5194,0.0670,0f000055,0*f00509a2\r\n#INSPVAXA,USB1,0,48.5,FINESTEERING,2089,274898.000,02000000,471d,15824;INS_SOLUTION_GOOD,INS_PSRSP,37.29129367359,127.14837394579,181.1256,23.4000,-0.0005,0.0027,-0.0016,0.570564156,0.405194685,245.326569333,0.8411,1.0183,1.5353,0.0013,0.0013,0.0011,0.5102,0.5194,0.0670,0f000055,0*0318aa58\r\n#INSPVAXA,USB1,0,48.0,FINESTEERING,2089,274898.500,02000000,471d,15824;INS_SOLUTION_GOOD,INS_PSRSP,37.29129332557,127.14837402134,181.1859,23.4000,0.0002,0.0031,-0.0021,0.567335093,0.406374938,245.335623784,0.8324,1.0112,1.5152,0.0013,0.0013,0.0011,0.5099,0.5192,0.0673,0f000045,0*5daafbc3\r\n#INSPVAXA,USB1,0,48.0,FINESTEERING,2089,274899.000,02000000,471d,15824;INS_SOLUTION_GOOD,INS_PSRSP,37.29129297382,127.14837410586,181.2468,23.4000,0.0002,0.0028,-0.0019,0.569279571,0.408142937,245.328968788,0.8324,1.0112,1.5152,0.0013,0.0013,0.0011,0.5099,0.5192,0.0673,0f000045,0*f1147de1\r\n#INSPVAXA,USB1,0,47.0,FINESTEERING,2089,274899.500,02000000,471d,15824;INS_SOLUTION_GOOD,INS_PSRSP,37.29129296082,127.14837409861,181.2492,23.4000,-0.0008,0.0012,-0.0011,0.569158681,0.406180048,245.333524723,0.8438,1.0206,1.5215,0.0013,0.0013,0.0011,0.5098,0.5191,0.0676,0f000044,0*9c0ee717\r\n#INSPVAXA,USB1,0,47.0,FINESTEERING,2089,274900.000,02000000,471d,15824;INS_SOLUTION_GOOD,INS_PSRSP,37.29129295686,127.14837408976,181.2494,23.4000,-0.0001,0.0006,-0.0024,0.567948756,0.404755086,245.334415668,0.8438,1.0206,1.5215,0.0013,0.0013,0.0011,0.5098,0.5191,0.0676,0f000044,0*ccc7197b\r\n#INSPVAXA,USB1,0,46.5,FINESTEERING,2089,274900.500,02000000,471d,15824;INS_SOLUTION_GOOD,INS_PSRSP,37.29129295660,127.14837408821,181.2497,23.4000,-0.0013,0.0001,-0.0022,0.563970177,0.400958630,245.333272980,0.8439,1.0207,1.5216,0.0013,0.0013,0.0011,0.5097,0.5191,0.0674,0f000054,0*508559bb\r\n#INSPVAXA,USB1,0,46.5,FINESTEERING,2089,274901.000,02000000,471d,15824;INS_SOLUTION_GOOD,INS_PSRSP,37.29129295588,127.14837408619,181.2497,23.4000,-0.0008,0.0000,-0.0013,0.563347585,0.400347208,245.330235090,0.8439,1.0207,1.5216,0.0013,0.0013,0.0011,0.5097,0.5191,0.0674,0f000054,0*7ec2af2d\r\n#INSPVAXA,USB1,0,46.5,FINESTEERING,2089,274901.500,02000000,471d,15824;INS_SOLUTION_GOOD,INS_PSRSP,37.29129296070,127.14837408609,181.2498,23.4000,-0.0007,0.0002,-0.0014,0.564699901,0.400306083,245.321341990,0.8440,1.0208,1.5216,0.0013,0.0013,0.0011,0.5096,0.5190,0.0672,0f000054,0*ce14039c\r\n#INSPVAXA,USB1,0,50.5,FINESTEERING,2089,274902.000,02000000,471d,15824;INS_SOLUTION_GOOD,INS_PSRSP,37.29129296495,127.14837408534,181.2497,23.4000,0.0004,-0.0002,-0.0011,0.564323701,0.400819389,245.315583259,0.8440,1.0208,1.5216,0.0013,0.0013,0.0011,0.5096,0.5190,0.0672,0f000054,0*2f4b2ec3\r\n#INSPVAXA,USB1,0,48.0,FINESTEERING,2089,274902.500,02000000,471d,15824;INS_SOLUTION_GOOD,INS_PSRSP,37.29129264850,127.14837416494,181.3031,23.4000,-0.0009,-0.0011,-0.0011,0.561483752,0.400418850,245.312109250,0.8248,1.0049,1.4965,0.0013,0.0013,0.0011,0.5095,0.5188,0.0668,0f000055,0*03135685\r\n#INSPVAXA,USB1,0,48.0,FINESTEERING,2089,274903.000,02000000,471d,15824;INS_SOLUTION_GOOD,INS_PSRSP,37.29129231506,127.14837424571,181.3590,23.4000,-0.0007,-0.0011,-0.0008,0.560973312,0.401788708,245.310689494,0.8248,1.0049,1.4965,0.0013,0.0013,0.0011,0.5095,0.5188,0.0668,0f000055,0*1b0655d7\r\n#INSPVAXA,USB1,0,48.0,FINESTEERING,2089,274903.500,02000000,471d,15824;INS_SOLUTION_GOOD,INS_PSRSP,37.29129202976,127.14837433545,181.4091,23.4000,-0.0010,0.0002,-0.0014,0.560156916,0.403120120,245.307691196,0.8176,0.9986,1.4787,0.0013,0.0013,0.0011,0.5094,0.5187,0.0665,0f000055,0*a87f3e02\r\n#INSPVAXA,USB1,0,48.0,FINESTEERING,2089,274904.000,02000000,471d,15824;INS_SOLUTION_GOOD,INS_PSRSP,37.29129173764,127.14837443072,181.4595,23.4000,-0.0018,0.0012,-0.0017,0.560624441,0.405387456,245.306996690,0.8176,0.9986,1.4787,0.0013,0.0013,0.0011,0.5094,0.5187,0.0665,0f000055,0*a067ff95\r\n#INSPVAXA,USB1,0,47.5,FINESTEERING,2089,274904.500,02000000,471d,15824;INS_SOLUTION_GOOD,INS_PSRSP,37.29129146978,127.14837450316,181.5066,23.4000,-0.0024,0.0003,-0.0017,0.559413620,0.406304298,245.301950912,0.8109,0.9928,1.4618,0.0013,0.0013,0.0011,0.5093,0.5187,0.0661,0f000055,0*6d6cb342\r\n#INSPVAXA,USB1,0,47.5,FINESTEERING,2089,274905.000,02000000,471d,15824;INS_SOLUTION_GOOD,INS_PSRSP,37.29129119398,127.14837457413,181.5542,23.4000,-0.0024,-0.0005,-0.0010,0.561495803,0.407839380,245.297287806,0.8109,0.9928,1.4618,0.0013,0.0013,0.0011,0.5093,0.5187,0.0661,0f000055,0*d4bbb853\r\n#INSPVAXA,USB1,0,47.5,FINESTEERING,2089,274905.500,02000000,471d,15824;INS_SOLUTION_GOOD,INS_PSRSP,37.29129094401,127.14837464509,181.5987,23.4000,-0.0030,-0.0004,-0.0010,0.562260195,0.409729883,245.297210916,0.8047,0.9871,1.4457,0.0013,0.0013,0.0011,0.5092,0.5186,0.0657,0f000055,0*8ed4d6c2\r\n#INSPVAXA,USB1,0,49.5,FINESTEERING,2089,274906.000,02000000,471d,15824;INS_SOLUTION_GOOD,INS_PSRSP,37.29129068354,127.14837471560,181.6439,23.4000,-0.0032,-0.0004,-0.0004,0.562606862,0.411286271,245.297439877,0.8047,0.9871,1.4457,0.0013,0.0013,0.0011,0.5092,0.5186,0.0657,0f000055,0*671d897a\r\n#INSPVAXA,USB1,0,48.0,FINESTEERING,2089,274906.500,02000000,471d,15824;INS_SOLUTION_GOOD,INS_PSRSP,37.29129045052,127.14837478514,181.6856,23.4000,-0.0022,-0.0002,-0.0004,0.565920365,0.413483722,245.292867558,0.7987,0.9817,1.4303,0.0013,0.0013,0.0011,0.5091,0.5184,0.0653,0f000055,0*dc6c1271\r\n#INSPVAXA,USB1,0,48.0,FINESTEERING,2089,274907.000,02000000,471d,15824;INS_SOLUTION_GOOD,INS_PSRSP,37.29129021052,127.14837485629,181.7276,23.4000,-0.0022,0.0001,-0.0016,0.567469179,0.414632976,245.288386791,0.7987,0.9817,1.4303,0.0013,0.0013,0.0011,0.5091,0.5184,0.0653,0f000055,0*f09fa4cb\r\n#INSPVAXA,USB1,0,46.5,FINESTEERING,2089,274907.500,02000000,471d,15824;INS_SOLUTION_GOOD,INS_PSRSP,37.29128999841,127.14837493238,181.7670,23.4000,-0.0009,0.0008,-0.0021,0.571577672,0.416317121,245.287668673,0.7931,0.9763,1.4156,0.0013,0.0013,0.0011,0.5090,0.5183,0.0649,0f000055,0*51588bc4\r\n#INSPVAXA,USB1,0,46.5,FINESTEERING,2089,274908.000,02000000,471d,15824;INS_SOLUTION_GOOD,INS_PSRSP,37.29128978452,127.14837501532,181.8065,23.4000,-0.0000,0.0019,-0.0019,0.574054122,0.415678550,245.283975944,0.7931,0.9763,1.4156,0.0013,0.0013,0.0011,0.5090,0.5183,0.0649,0f000055,0*d8928a45\r\n#INSPVAXA,USB1,0,46.5,FINESTEERING,2089,274908.500,02000000,471d,15824;INS_SOLUTION_GOOD,INS_PSRSP,37.29128957870,127.14837508440,181.8447,23.4000,0.0002,0.0014,-0.0011,0.575177058,0.415711262,245.285612068,0.7877,0.9712,1.4015,0.0013,0.0013,0.0011,0.5089,0.5183,0.0645,0f000055,0*2e42c43c\r\n#INSPVAXA,USB1,0,50.0,FINESTEERING,2089,274909.000,02000000,471d,15824;INS_SOLUTION_GOOD,INS_PSRSP,37.29128936878,127.14837515415,181.8832,23.4000,-0.0009,0.0012,-0.0012,0.573130107,0.415427095,245.290124097,0.7877,0.9712,1.4015,0.0013,0.0013,0.0011,0.5089,0.5183,0.0645,0f000055,0*e9b68213\r\n#INSPVAXA,USB1,0,48.0,FINESTEERING,2089,274909.500,02000000,471d,15824;INS_SOLUTION_GOOD,INS_PSRSP,37.29128917943,127.14837522011,181.9192,23.4000,0.0005,0.0010,-0.0012,0.573726211,0.415850403,245.288307202,0.7827,0.9663,1.3881,0.0013,0.0013,0.0011,0.5089,0.5182,0.0640,0f000055,0*034ca210\r\n#INSPVAXA,USB1,0,48.0,FINESTEERING,2089,274910.000,02000000,471d,15824;INS_SOLUTION_GOOD,INS_PSRSP,37.29128898803,127.14837528888,181.9555,23.4000,0.0013,0.0012,-0.0008,0.576780808,0.416141692,245.292672735,0.7827,0.9663,1.3881,0.0013,0.0013,0.0011,0.5089,0.5182,0.0640,0f000055,0*09b56bfa\r\n#INSPVAXA,USB1,0,48.0,FINESTEERING,2089,274910.500,02000000,471d,15824;INS_SOLUTION_GOOD,INS_PSRSP,37.29128879984,127.14837535394,181.9907,23.4000,0.0002,0.0009,-0.0003,0.576605890,0.415055112,245.290848171,0.7779,0.9616,1.3752,0.0013,0.0013,0.0011,0.5088,0.5181,0.0635,0f000055,0*6bd502db\r\n#INSPVAXA,USB1,0,50.0,FINESTEERING,2089,274911.000,02000000,471d,15824;INS_SOLUTION_GOOD,INS_PSRSP,37.29128860937,127.14837541975,182.0262,23.4000,-0.0007,0.0007,-0.0001,0.574652372,0.415001376,245.285214067,0.7779,0.9616,1.3752,0.0013,0.0013,0.0011,0.5088,0.5181,0.0635,0f000055,0*3232dd27\r\n#INSPVAXA,USB1,0,50.0,FINESTEERING,2089,274911.500,02000000,471d,15824;INS_SOLUTION_GOOD,INS_PSRSP,37.29128843304,127.14837547918,182.0592,23.4000,-0.0014,-0.0002,-0.0011,0.572440821,0.414251657,245.283646236,0.7733,0.9570,1.3628,0.0013,0.0013,0.0011,0.5087,0.5179,0.0630,0f000055,0*e2708a46\r\n#INSPVAXA,USB1,0,50.0,FINESTEERING,2089,274912.000,02000000,471d,15824;INS_SOLUTION_GOOD,INS_PSRSP,37.29128825101,127.14837553962,182.0923,23.4000,-0.0014,0.0005,-0.0014,0.571994230,0.413398467,245.284461100,0.7733,0.9570,1.3628,0.0013,0.0013,0.0011,0.5087,0.5179,0.0630,0f000055,0*83b383f1\r\n#INSPVAXA,USB1,0,48.0,FINESTEERING,2089,274912.500,02000000,471d,15824;INS_SOLUTION_GOOD,INS_PSRSP,37.29128807989,127.14837560036,182.1249,23.4000,-0.0020,0.0004,-0.0015,0.571511814,0.413096776,245.283154220,0.7688,0.9524,1.3509,0.0013,0.0013,0.0011,0.5086,0.5178,0.0626,0f000055,0*95555e7f\r\n#INSPVAXA,USB1,0,48.0,FINESTEERING,2089,274913.000,02000000,471d,15824;INS_SOLUTION_GOOD,INS_PSRSP,37.29128789890,127.14837566342,182.1578,23.4000,-0.0032,0.0007,-0.0014,0.571681287,0.414381102,245.281138052,0.7688,0.9524,1.3509,0.0013,0.0013,0.0011,0.5086,0.5178,0.0626,0f000055,0*660b4c74\r\n#INSPVAXA,USB1,0,48.0,FINESTEERING,2089,274913.500,02000000,471d,15824;INS_SOLUTION_GOOD,INS_PSRSP,37.29128773350,127.14837572073,182.1887,23.4000,-0.0041,0.0012,-0.0009,0.575159017,0.416035188,245.280968285,0.7644,0.9480,1.3394,0.0013,0.0013,0.0011,0.5085,0.5177,0.0622,0f000055,0*23c3313a\r\n#INSPVAXA,USB1,0,51.0,FINESTEERING,2089,274914.000,02000000,471d,15824;INS_SOLUTION_GOOD,INS_PSRSP,37.29128755782,127.14837578248,182.2201,23.4000,-0.0044,0.0012,-0.0005,0.578733472,0.415761447,245.276510942,0.7644,0.9480,1.3394,0.0013,0.0013,0.0011,0.5085,0.5177,0.0622,0f000055,0*e95f1a05\r\n#INSPVAXA,USB1,0,50.0,FINESTEERING,2089,274914.500,02000000,471d,15824;INS_SOLUTION_GOOD,INS_PSRSP,37.29128740960,127.14837583085,182.2498,23.4000,-0.0028,0.0007,-0.0002,0.583171521,0.415305355,245.277140673,0.7602,0.9436,1.3283,0.0013,0.0013,0.0011,0.5084,0.5175,0.0618,0f000055,0*53603f08\r\n#INSPVAXA,USB1,0,50.0,FINESTEERING,2089,274915.000,02000000,471d,15824;INS_SOLUTION_GOOD,INS_PSRSP,37.29128725675,127.14837587973,182.2798,23.4000,-0.0025,0.0004,-0.0004,0.587620310,0.415842385,245.273740711,0.7602,0.9436,1.3283,0.0013,0.0013,0.0011,0.5084,0.5175,0.0618,0f000055,0*69cc6b82\r\n#INSPVAXA,USB1,0,50.0,FINESTEERING,2089,274915.500,02000000,471d,15824;INS_SOLUTION_GOOD,INS_PSRSP,37.29128711458,127.14837592824,182.3076,23.4000,-0.0013,0.0001,-0.0012,0.593788867,0.417165062,245.275764696,0.7562,0.9393,1.3176,0.0013,0.0013,0.0011,0.5083,0.5174,0.0614,0f000055,0*d94d48e6\r\n#INSPVAXA,USB1,0,50.0,FINESTEERING,2089,274916.000,02000000,471d,15824;INS_SOLUTION_GOOD,INS_PSRSP,37.29128697257,127.14837597765,182.3355,23.4000,0.0010,0.0004,-0.0025,0.600386514,0.416649142,245.268477625,0.7562,0.9393,1.3176,0.0013,0.0013,0.0011,0.5083,0.5174,0.0614,0f000055,0*2350fbfb\r\n#INSPVAXA,USB1,0,50.0,FINESTEERING,2089,274916.500,02000000,471d,15824;INS_SOLUTION_GOOD,INS_PSRSP,37.29128683384,127.14837602374,182.3631,23.4000,0.0009,-0.0002,-0.0016,0.601576356,0.417752369,245.261171067,0.7523,0.9352,1.3073,0.0013,0.0013,0.0011,0.5082,0.5174,0.0611,0f000055,0*0f9b4284\r\n#INSPVAXA,USB1,0,50.5,FINESTEERING,2089,274917.000,02000000,471d,15824;INS_SOLUTION_GOOD,INS_PSRSP,37.29128669472,127.14837606957,182.3908,23.4000,0.0007,-0.0005,-0.0014,0.598832961,0.417793483,245.257951842,0.7523,0.9352,1.3073,0.0013,0.0013,0.0011,0.5082,0.5174,0.0611,0f000055,0*991b17db\r\n#INSPVAXA,USB1,0,50.5,FINESTEERING,2089,274917.500,02000000,471d,15824;INS_SOLUTION_GOOD,INS_PSRSP,37.29128656308,127.14837611782,182.4168,23.4000,0.0007,0.0003,-0.0013,0.600994925,0.419398156,245.259682056,0.7485,0.9311,1.2973,0.0013,0.0013,0.0011,0.5082,0.5172,0.0610,0f000055,0*fe30a799\r\n#INSPVAXA,USB1,0,50.5,FINESTEERING,2089,274918.000,02000000,471d,15824;INS_SOLUTION_GOOD,INS_PSRSP,37.29128643141,127.14837617087,182.4432,23.4000,0.0013,0.0012,-0.0010,0.600460436,0.420691872,245.259764897,0.7485,0.9311,1.2973,0.0013,0.0013,0.0011,0.5082,0.5172,0.0610,0f000055,0*b3528053\r\n#INSPVAXA,USB1,0,49.0,FINESTEERING,2089,274918.500,02000000,471d,15824;INS_SOLUTION_GOOD,INS_PSRSP,37.29128630423,127.14837621349,182.4682,23.4000,0.0005,0.0006,-0.0006,0.601762536,0.418603304,245.256248529,0.7449,0.9271,1.2877,0.0013,0.0013,0.0011,0.5080,0.5171,0.0609,0f000055,0*878c4a7d\r\n#INSPVAXA,USB1,0,49.0,FINESTEERING,2089,274919.000,02000000,471d,15824;INS_SOLUTION_GOOD,INS_PSRSP,37.29128617448,127.14837625271,182.4936,23.4000,0.0004,-0.0009,-0.0001,0.602909920,0.417368346,245.253650200,0.7449,0.9271,1.2877,0.0013,0.0013,0.0011,0.5080,0.5171,0.0609,0f000055,0*641aa3f6\r\n#INSPVAXA,USB1,0,49.0,FINESTEERING,2089,274919.500,02000000,471d,15824;INS_SOLUTION_GOOD,INS_PSRSP,37.29128605618,127.14837629505,182.5173,23.4000,0.0005,-0.0002,0.0000,0.604052974,0.419235841,245.251924396,0.7413,0.9233,1.2784,0.0013,0.0013,0.0011,0.5079,0.5169,0.0607,0f000055,0*13e32e00\r\n#INSPVAXA,USB1,0,52.0,FINESTEERING,2089,274920.000,02000000,471d,15824;INS_SOLUTION_GOOD,INS_PSRSP,37.29128593914,127.14837633840,182.5412,23.4000,0.0012,0.0002,-0.0006,0.605808632,0.418930547,245.247730652,0.7413,0.9233,1.2784,0.0013,0.0013,0.0011,0.5079,0.5169,0.0607,0f000055,0*8249896b\r\n#INSPVAXA,USB1,0,50.5,FINESTEERING,2089,274920.500,02000000,471d,15824;INS_SOLUTION_GOOD,INS_PSRSP,37.29128582889,127.14837637651,182.5636,23.4000,0.0013,0.0001,-0.0008,0.607806892,0.417532906,245.242927817,0.7379,0.9195,1.2694,0.0013,0.0013,0.0011,0.5078,0.5168,0.0605,0f000055,0*e8d244d9\r\n#INSPVAXA,USB1,0,50.5,FINESTEERING,2089,274921.000,02000000,471d,15824;INS_SOLUTION_GOOD,INS_PSRSP,37.29128572131,127.14837641473,182.5861,23.4000,0.0027,-0.0006,-0.0013,0.606792671,0.417450131,245.241520551,0.7379,0.9195,1.2694,0.0013,0.0013,0.0011,0.5078,0.5168,0.0605,0f000055,0*ab9c3c42\r\n#INSPVAXA,USB1,0,50.5,FINESTEERING,2089,274921.500,02000000,471d,15824;INS_SOLUTION_GOOD,INS_PSRSP,37.29128582704,127.14837645596,182.5692,23.4000,0.0027,-0.0010,-0.0007,0.608615432,0.416830374,245.243001745,0.7334,0.9157,1.2589,0.0013,0.0013,0.0011,0.5077,0.5167,0.0603,0f000055,0*56c60759\r\n#INSPVAXA,USB1,0,50.5,FINESTEERING,2089,274922.000,02000000,471d,15824;INS_SOLUTION_GOOD,INS_PSRSP,37.29128594586,127.14837649318,182.5506,23.4000,0.0032,-0.0013,-0.0003,0.609374482,0.416377668,245.243848604,0.7334,0.9157,1.2589,0.0013,0.0013,0.0011,0.5077,0.5167,0.0603,0f000055,0*778b6419\r\n#INSPVAXA,USB1,0,50.5,FINESTEERING,2089,274922.500,02000000,471d,15824;INS_SOLUTION_GOOD,INS_PSRSP,37.29128605008,127.14837653863,182.5326,23.4000,0.0027,-0.0003,-0.0001,0.607059437,0.415084031,245.242122466,0.7292,0.9120,1.2487,0.0013,0.0013,0.0011,0.5076,0.5166,0.0600,0f000055,0*6f990815\r\n#INSPVAXA,USB1,0,51.0,FINESTEERING,2089,274923.000,02000000,471d,15824;INS_SOLUTION_GOOD,INS_PSRSP,37.29128615764,127.14837658679,182.5145,23.4000,0.0016,0.0005,0.0001,0.605895585,0.414267409,245.241985978,0.7292,0.9120,1.2487,0.0013,0.0013,0.0011,0.5076,0.5166,0.0600,0f000055,0*64d01127\r\n#INSPVAXA,USB1,0,51.0,FINESTEERING,2089,274923.500,02000000,471d,15824;INS_SOLUTION_GOOD,INS_PSRSP,37.29128627128,127.14837663753,182.4968,23.4000,0.0010,-0.0001,0.0006,0.607265596,0.414710443,245.243551317,0.7250,0.9084,1.2390,0.0013,0.0013,0.0011,0.5075,0.5164,0.0598,0f000055,0*05f671fe\r\n#INSPVAXA,USB1,0,51.0,FINESTEERING,2089,274924.000,02000000,471d,15824;INS_SOLUTION_GOOD,INS_PSRSP,37.29128638457,127.14837668495,182.4791,23.4000,-0.0001,-0.0009,0.0016,0.605739290,0.413719144,245.242356946,0.7250,0.9084,1.2390,0.0013,0.0013,0.0011,0.5075,0.5164,0.0598,0f000055,0*7862ebfb\r\n#INSPVAXA,USB1,0,48.0,FINESTEERING,2089,274924.500,02000000,471d,15824;INS_SOLUTION_GOOD,INS_PSRSP,37.29128649489,127.14837673724,182.4617,23.4000,0.0004,-0.0003,0.0018,0.606848324,0.415325470,245.241495932,0.7210,0.9048,1.2295,0.0013,0.0013,0.0011,0.5074,0.5163,0.0595,0f000055,0*8c4d300e\r\n#INSPVAXA,USB1,0,48.0,FINESTEERING,2089,274925.000,02000000,471d,15824;INS_SOLUTION_GOOD,INS_PSRSP,37.29128661278,127.14837678895,182.4442,23.4000,0.0024,-0.0005,0.0014,0.607588296,0.416071514,245.240999205,0.7210,0.9048,1.2295,0.0013,0.0013,0.0011,0.5074,0.5163,0.0595,0f000055,0*93b87b6b\r\n#INSPVAXA,USB1,0,48.0,FINESTEERING,2089,274925.500,02000000,471d,15824;INS_SOLUTION_GOOD,INS_PSRSP,37.29128671783,127.14837684121,182.4272,23.4000,0.0016,0.0002,0.0009,0.605335678,0.417340060,245.242840044,0.7171,0.9012,1.2203,0.0013,0.0013,0.0011,0.5073,0.5162,0.0591,0f000055,0*e37714ea\r\n#INSPVAXA,USB1,0,48.0,FINESTEERING,2089,274926.000,02000000,471d,15824;INS_SOLUTION_GOOD,INS_PSRSP,37.29128682925,127.14837689730,182.4098,23.4000,0.0026,0.0006,-0.0000,0.605330972,0.416518668,245.242446570,0.7171,0.9012,1.2203,0.0013,0.0013,0.0011,0.5073,0.5162,0.0591,0f000055,0*d9f7d8ff\r\n#INSPVAXA,USB1,0,48.0,FINESTEERING,2089,274926.500,02000000,471d,15824;INS_SOLUTION_GOOD,INS_PSRSP,37.29128692956,127.14837694480,182.3934,23.4000,0.0025,-0.0002,-0.0002,0.603467825,0.414973408,245.242951277,0.7132,0.8976,1.2114,0.0012,0.0012,0.0011,0.5072,0.5161,0.0588,0f000055,0*e2be8341\r\n#INSPVAXA,USB1,0,49.5,FINESTEERING,2089,274927.000,02000000,471d,15824;INS_SOLUTION_GOOD,INS_PSRSP,37.29128703409,127.14837699088,182.3768,23.4000,0.0018,-0.0006,-0.0003,0.604146839,0.412556254,245.241970256,0.7132,0.8976,1.2114,0.0012,0.0012,0.0011,0.5072,0.5161,0.0588,0f000055,0*e184bd5e\r\n#INSPVAXA,USB1,0,49.5,FINESTEERING,2089,274927.500,02000000,471d,15824;INS_SOLUTION_GOOD,INS_PSRSP,37.29128712285,127.14837704351,182.3613,23.4000,0.0011,-0.0005,-0.0004,0.604858828,0.412691310,245.239605822,0.7095,0.8940,1.2028,0.0012,0.0012,0.0011,0.5072,0.5160,0.0584,0f000055,0*fa37ad25\r\n#INSPVAXA,USB1,0,51.0,FINESTEERING,2089,274928.000,02000000,471d,15824;INS_SOLUTION_GOOD,INS_PSRSP,37.29128721376,127.14837709381,182.3455,23.4000,0.0002,-0.0008,-0.0003,0.605238455,0.411602789,245.240256836,0.7095,0.8940,1.2028,0.0012,0.0012,0.0011,0.5072,0.5160,0.0584,0f000055,0*51aa4d34\r\n#INSPVAXA,USB1,0,48.5,FINESTEERING,2089,274928.500,02000000,471d,15824;INS_SOLUTION_GOOD,INS_PSRSP,37.29128730711,127.14837714520,182.3306,23.4000,0.0017,-0.0011,-0.0004,0.608084035,0.412753895,245.239310014,0.7058,0.8904,1.1944,0.0012,0.0012,0.0011,0.5071,0.5159,0.0581,0f000055,0*04945f4e\r\n#INSPVAXA,USB1,0,48.5,FINESTEERING,2089,274929.000,02000000,471d,15824;INS_SOLUTION_GOOD,INS_PSRSP,37.29128740638,127.14837719537,182.3154,23.4000,0.0028,-0.0007,-0.0003,0.609275742,0.413660694,245.238526305,0.7058,0.8904,1.1944,0.0012,0.0012,0.0011,0.5071,0.5159,0.0581,0f000055,0*b839a0d2\r\n#INSPVAXA,USB1,0,48.5,FINESTEERING,2089,274929.500,02000000,471d,15824;INS_SOLUTION_GOOD,INS_PSRSP,37.29128748440,127.14837722996,182.3019,23.4000,0.0030,-0.0007,-0.0004,0.608035595,0.412531391,245.237789046,0.7021,0.8869,1.1862,0.0012,0.0012,0.0011,0.5070,0.5159,0.0579,0f000055,0*21dd3410\r\n#INSPVAXA,USB1,0,49.5,FINESTEERING,2089,274930.000,02000000,471d,15824;INS_SOLUTION_GOOD,INS_PSRSP,37.29128757008,127.14837726275,182.2878,23.4000,0.0028,-0.0009,-0.0010,0.607586790,0.410488911,245.240042124,0.7021,0.8869,1.1862,0.0012,0.0012,0.0011,0.5070,0.5159,0.0579,0f000055,0*b0ac66fd\r\n#INSPVAXA,USB1,0,47.5,FINESTEERING,2089,274930.500,02000000,471d,15824;INS_SOLUTION_GOOD,INS_PSRSP,37.29128764428,127.14837729525,182.2743,23.4000,0.0026,-0.0007,-0.0018,0.610281676,0.410696764,245.236778200,0.6985,0.8833,1.1782,0.0013,0.0013,0.0011,0.5069,0.5158,0.0577,0f000055,0*87a30cab\r\n#INSPVAXA,USB1,0,47.5,FINESTEERING,2089,274931.000,02000000,471d,15824;INS_SOLUTION_GOOD,INS_PSRSP,37.29128772160,127.14837732534,182.2602,23.4000,0.0015,-0.0014,-0.0022,0.609024731,0.410441075,245.238981565,0.6985,0.8833,1.1782,0.0013,0.0013,0.0011,0.5069,0.5158,0.0577,0f000055,0*37a8765d\r\n#INSPVAXA,USB1,0,47.5,FINESTEERING,2089,274931.500,02000000,471d,15824;INS_SOLUTION_GOOD,INS_PSRSP,37.29128779035,127.14837735276,182.2478,23.4000,0.0005,-0.0022,-0.0019,0.609944312,0.412117678,245.239289970,0.6950,0.8797,1.1704,0.0013,0.0013,0.0011,0.5069,0.5157,0.0575,0f000055,0*0adc938e\r\n#INSPVAXA,USB1,0,50.0,FINESTEERING,2089,274932.000,02000000,471d,15824;INS_SOLUTION_GOOD,INS_PSRSP,37.29128786009,127.14837737031,182.2351,23.4000,-0.0000,-0.0038,-0.0010,0.609815093,0.413595550,245.238390468,0.6950,0.8797,1.1704,0.0013,0.0013,0.0011,0.5069,0.5157,0.0575,0f000055,0*8566ff58\r\n#INSPVAXA,USB1,0,50.0,FINESTEERING,2089,274932.500,02000000,471d,15824;INS_SOLUTION_GOOD,INS_PSRSP,37.29128794509,127.14837755795,182.2196,23.4000,0.0016,-0.0021,-0.0016,0.611068342,0.417739750,245.237316659,0.6914,0.8761,1.1628,0.0013,0.0013,0.0011,0.5068,0.5156,0.0573,0f000055,0*a9a8bde6\r\n#INSPVAXA,USB1,0,50.5,FINESTEERING,2089,274933.000,02000000,471d,15824;INS_SOLUTION_GOOD,INS_PSRSP,37.29128803718,127.14837774891,182.2032,23.4000,0.0029,-0.0017,-0.0021,0.609280729,0.421134643,245.239034475,0.6914,0.8761,1.1628,0.0013,0.0013,0.0011,0.5068,0.5156,0.0573,0f000055,0*fcff294c\r\n#INSPVAXA,USB1,0,50.0,FINESTEERING,2089,274933.500,02000000,471d,15824;INS_SOLUTION_GOOD,INS_PSRSP,37.29128811116,127.14837792727,182.1881,23.4000,0.0017,-0.0022,-0.0013,0.609057507,0.419747636,245.238570763,0.6880,0.8725,1.1554,0.0012,0.0012,0.0011,0.5067,0.5156,0.0570,0f000055,0*1a13d35c\r\n#INSPVAXA,USB1,0,50.0,FINESTEERING,2089,274934.000,02000000,471d,15824;INS_SOLUTION_GOOD,INS_PSRSP,37.29128818687,127.14837809844,182.1729,23.4000,0.0014,-0.0030,-0.0005,0.607208446,0.420337408,245.235956718,0.6880,0.8725,1.1554,0.0012,0.0012,0.0011,0.5067,0.5156,0.0570,0f000055,0*91e4ff3d\r\n#INSPVAXA,USB1,0,47.5,FINESTEERING,2089,274934.500,02000000,471d,15824;INS_SOLUTION_GOOD,INS_PSRSP,37.29128826540,127.14837827633,182.1586,23.4000,0.0022,-0.0021,0.0000,0.604391575,0.423213787,245.233791883,0.6846,0.8690,1.1481,0.0013,0.0013,0.0011,0.5065,0.5154,0.0569,0f000055,0*98406f26\r\n#INSPVAXA,USB1,0,47.5,FINESTEERING,2089,274935.000,02000000,471d,15824;INS_SOLUTION_GOOD,INS_PSRSP,37.29128835017,127.14837845380,182.1438,23.4000,0.0023,-0.0018,-0.0001,0.600239632,0.424403694,245.235580503,0.6846,0.8690,1.1481,0.0013,0.0013,0.0011,0.5065,0.5154,0.0569,0f000055,0*4548d212\r\n#INSPVAXA,USB1,0,47.5,FINESTEERING,2089,274935.500,02000000,471d,15824;INS_SOLUTION_GOOD,INS_PSRSP,37.29128842136,127.14837862395,182.1293,23.4000,0.0027,-0.0008,-0.0005,0.599175730,0.424611138,245.233431218,0.6813,0.8654,1.1411,0.0013,0.0013,0.0011,0.5064,0.5153,0.0570,0f000055,0*21941805\r\n#INSPVAXA,USB1,0,48.5,FINESTEERING,2089,274936.000,02000000,471d,15824;INS_SOLUTION_GOOD,INS_PSRSP,37.29128849870,127.14837879495,182.1144,23.4000,0.0032,-0.0009,-0.0010,0.596607144,0.423625385,245.235853635,0.6813,0.8654,1.1411,0.0013,0.0013,0.0011,0.5064,0.5153,0.0570,0f000055,0*737bd2fa\r\n#INSPVAXA,USB1,0,45.0,FINESTEERING,2089,274936.500,02000000,471d,15824;INS_SOLUTION_GOOD,INS_PSRSP,37.29128856418,127.14837895387,182.1006,23.4000,0.0018,-0.0016,-0.0008,0.597031431,0.423937024,245.235562446,0.6780,0.8619,1.1341,0.0013,0.0013,0.0011,0.5064,0.5152,0.0570,0f000055,0*528c3b02\r\n#INSPVAXA,USB1,0,45.0,FINESTEERING,2089,274937.000,02000000,471d,15824;INS_SOLUTION_GOOD,INS_PSRSP,37.29128863263,127.14837910612,182.0866,23.4000,0.0012,-0.0031,-0.0005,0.595190679,0.421395188,245.236230459,0.6780,0.8619,1.1341,0.0013,0.0013,0.0011,0.5064,0.5152,0.0570,0f000055,0*d7c76431\r\n#INSPVAXA,USB1,0,45.0,FINESTEERING,2089,274937.500,02000000,471d,15824;INS_SOLUTION_GOOD,INS_PSRSP,37.29128869993,127.14837926366,182.0737,23.4000,0.0011,-0.0030,0.0003,0.593968709,0.426322912,245.239903863,0.6747,0.8584,1.1274,0.0013,0.0013,0.0011,0.5062,0.5151,0.0569,0f000055,0*8af9427d\r\n#INSPVAXA,USB1,0,48.5,FINESTEERING,2089,274938.000,02000000,471d,15824;INS_SOLUTION_GOOD,INS_PSRSP,37.29128877279,127.14837942149,182.0608,23.4000,0.0017,-0.0018,0.0007,0.593606818,0.427897722,245.237777753,0.6747,0.8584,1.1274,0.0013,0.0013,0.0011,0.5062,0.5151,0.0569,0f000055,0*7bf5cf45\r\n#INSPVAXA,USB1,0,48.5,FINESTEERING,2089,274938.500,02000000,471d,15824;INS_SOLUTION_GOOD,INS_PSRSP,37.29128883766,127.14837957935,182.0476,23.4000,0.0012,-0.0010,-0.0002,0.592336251,0.428107065,245.235914543,0.6715,0.8549,1.1207,0.0013,0.0013,0.0011,0.5061,0.5150,0.0569,0f000055,0*c3c39170\r\n#INSPVAXA,USB1,0,49.5,FINESTEERING,2089,274939.000,02000000,471d,15824;INS_SOLUTION_GOOD,INS_PSRSP,37.29128890550,127.14837973923,182.0342,23.4000,0.0010,-0.0001,-0.0003,0.592526442,0.427745946,245.234229964,0.6715,0.8549,1.1207,0.0013,0.0013,0.0011,0.5061,0.5150,0.0569,0f000055,0*48e0603b\r\n#INSPVAXA,USB1,0,48.5,FINESTEERING,2089,274939.500,02000000,471d,15824;INS_SOLUTION_GOOD,INS_PSRSP,37.29128896654,127.14837988841,182.0219,23.4000,0.0010,0.0004,-0.0001,0.592554769,0.427563708,245.231632593,0.6682,0.8514,1.1142,0.0013,0.0013,0.0011,0.5060,0.5149,0.0570,0f000055,0*dd89fb48\r\n#INSPVAXA,USB1,0,48.5,FINESTEERING,2089,274940.000,02000000,471d,15824;INS_SOLUTION_GOOD,INS_PSRSP,37.29128903295,127.14838004010,182.0092,23.4000,0.0022,-0.0001,-0.0004,0.590678653,0.426804742,245.228442585,0.6682,0.8514,1.1142,0.0013,0.0013,0.0011,0.5060,0.5149,0.0570,0f000055,0*2c8fedfa\r\n#INSPVAXA,USB1,0,48.5,FINESTEERING,2089,274940.500,02000000,471d,15824;INS_SOLUTION_GOOD,INS_PSRSP,37.29128909661,127.14838017571,181.9972,23.4000,0.0017,0.0002,-0.0006,0.587255571,0.426204575,245.225106885,0.6650,0.8479,1.1078,0.0013,0.0013,0.0011,0.5059,0.5148,0.0575,0f000055,0*b166285e\r\n#INSPVAXA,USB1,0,52.5,FINESTEERING,2089,274941.000,02000000,471d,15824;INS_SOLUTION_GOOD,INS_PSRSP,37.29128916541,127.14838031322,181.9849,23.4000,0.0021,-0.0002,-0.0005,0.584224631,0.423781472,245.222018230,0.6650,0.8479,1.1078,0.0013,0.0013,0.0011,0.5059,0.5148,0.0575,0f000055,0*d99fe873\r\n#INSPVAXA,USB1,0,48.5,FINESTEERING,2089,274941.500,02000000,471d,15824;INS_SOLUTION_GOOD,INS_PSRSP,37.29128922552,127.14838044293,181.9738,23.4000,0.0012,0.0003,-0.0002,0.582139644,0.424200200,245.223639910,0.6618,0.8444,1.1015,0.0013,0.0013,0.0011,0.5059,0.5147,0.0581,0f000055,0*ef9c769c\r\n#INSPVAXA,USB1,0,48.5,FINESTEERING,2089,274942.000,02000000,471d,15824;INS_SOLUTION_GOOD,INS_PSRSP,37.29128928501,127.14838057225,181.9624,23.4000,-0.0003,-0.0008,-0.0006,0.580345932,0.423133808,245.222481229,0.6618,0.8444,1.1015,0.0013,0.0013,0.0011,0.5059,0.5147,0.0581,0f000055,0*86e47425\r\n#INSPVAXA,USB1,0,47.0,FINESTEERING,2089,274942.500,02000000,471d,15824;INS_SOLUTION_GOOD,INS_PSRSP,37.29128934483,127.14838069296,181.9516,23.4000,-0.0001,-0.0021,-0.0004,0.582288197,0.424996386,245.222449475,0.6586,0.8408,1.0953,0.0013,0.0013,0.0011,0.5058,0.5147,0.0585,0f000055,0*2830876c\r\n#INSPVAXA,USB1,0,47.0,FINESTEERING,2089,274943.000,02000000,471d,15824;INS_SOLUTION_GOOD,INS_PSRSP,37.29128940802,127.14838080698,181.9404,23.4000,0.0000,-0.0029,-0.0004,0.583300081,0.428287757,245.222255206,0.6586,0.8408,1.0953,0.0013,0.0013,0.0011,0.5058,0.5147,0.0585,0f000055,0*080e610f\r\n#INSPVAXA,USB1,0,47.0,FINESTEERING,2089,274943.500,02000000,471d,15824;INS_SOLUTION_GOOD,INS_PSRSP,37.29128947168,127.14838093031,181.9295,23.4000,0.0011,-0.0016,-0.0003,0.581705820,0.432509763,245.220625056,0.6554,0.8373,1.0892,0.0013,0.0013,0.0011,0.5056,0.5146,0.0589,0f000055,0*396b230f\r\n#INSPVAXA,USB1,0,49.5,FINESTEERING,2089,274944.000,02000000,471d,15824;INS_SOLUTION_GOOD,INS_PSRSP,37.29128954172,127.14838105538,181.9185,23.4000,0.0028,-0.0001,-0.0007,0.582005582,0.436607595,245.223109822,0.6554,0.8373,1.0892,0.0013,0.0013,0.0011,0.5056,0.5146,0.0589,0f000055,0*3eb619c2\r\n#INSPVAXA,USB1,0,49.5,FINESTEERING,2089,274944.500,02000000,471d,15824;INS_SOLUTION_GOOD,INS_PSRSP,37.29128959709,127.14838117634,181.9081,23.4000,0.0021,0.0002,-0.0009,0.584119207,0.435603974,245.219909515,0.6523,0.8338,1.0831,0.0013,0.0013,0.0011,0.5055,0.5144,0.0591,0f000055,0*a5ce1914\r\n#INSPVAXA,USB1,0,49.5,FINESTEERING,2089,274945.000,02000000,471d,15824;INS_SOLUTION_GOOD,INS_PSRSP,37.29128965420,127.14838129714,181.8973,23.4000,0.0010,0.0001,-0.0013,0.580870180,0.435144654,245.216556355,0.6523,0.8338,1.0831,0.0013,0.0013,0.0011,0.5055,0.5144,0.0591,0f000055,0*77b0fe78\r\n#INSPVAXA,USB1,0,49.5,FINESTEERING,2089,274945.500,02000000,471d,15824;INS_SOLUTION_GOOD,INS_PSRSP,37.29128970897,127.14838140908,181.8873,23.4000,0.0014,0.0006,-0.0013,0.579515179,0.436208023,245.215920816,0.6492,0.8303,1.0773,0.0013,0.0013,0.0011,0.5055,0.5144,0.0593,0f000055,0*59d1c280\r\n#INSPVAXA,USB1,0,49.5,FINESTEERING,2089,274946.000,02000000,471d,15824;INS_SOLUTION_GOOD,INS_PSRSP,37.29128977038,127.14838152677,181.8769,23.4000,0.0028,0.0014,-0.0013,0.577882656,0.436813713,245.212084526,0.6492,0.8303,1.0773,0.0013,0.0013,0.0011,0.5055,0.5144,0.0593,0f000055,0*c143565a\r\n#INSPVAXA,USB1,0,49.5,FINESTEERING,2089,274946.500,02000000,471d,15824;INS_SOLUTION_GOOD,INS_PSRSP,37.29128982294,127.14838162842,181.8671,23.4000,0.0012,0.0007,-0.0014,0.575482306,0.435561817,245.210251409,0.6462,0.8269,1.0715,0.0013,0.0013,0.0011,0.5054,0.5143,0.0595,0f000055,0*590b6eec\r\n#INSPVAXA,USB1,0,49.5,FINESTEERING,2089,274947.000,02000000,471d,15824;INS_SOLUTION_GOOD,INS_PSRSP,37.29128987870,127.14838172966,181.8567,23.4000,0.0012,-0.0004,-0.0022,0.574285929,0.431953750,245.206836959,0.6462,0.8269,1.0715,0.0013,0.0013,0.0011,0.5054,0.5143,0.0595,0f000055,0*9926b46d\r\n#INSPVAXA,USB1,0,49.5,FINESTEERING,2089,274947.500,02000000,471d,15824;INS_SOLUTION_GOOD,INS_PSRSP,37.29128993404,127.14838182944,181.8476,23.4000,0.0018,-0.0010,-0.0015,0.575090804,0.432714944,245.204773701,0.6431,0.8235,1.0658,0.0013,0.0013,0.0011,0.5053,0.5142,0.0596,0f000055,0*cdeb5998\r\n#INSPVAXA,USB1,0,51.5,FINESTEERING,2089,274948.000,02000000,471d,15824;INS_SOLUTION_GOOD,INS_PSRSP,37.29128999354,127.14838192772,181.8384,23.4000,0.0018,-0.0012,-0.0003,0.574022786,0.434657432,245.203426479,0.6431,0.8235,1.0658,0.0013,0.0013,0.0011,0.5053,0.5142,0.0596,0f000055,0*98f0b478\r\n#INSPVAXA,USB1,0,49.5,FINESTEERING,2089,274948.500,02000000,471d,15824;INS_SOLUTION_GOOD,INS_PSRSP,37.29129004679,127.14838203067,181.8292,23.4000,0.0027,0.0006,-0.0009,0.573436151,0.436105214,245.201969916,0.6401,0.8201,1.0602,0.0013,0.0013,0.0011,0.5052,0.5141,0.0597,0f000055,0*049fcf24\r\n#INSPVAXA,USB1,0,49.5,FINESTEERING,2089,274949.000,02000000,471d,15824;INS_SOLUTION_GOOD,INS_PSRSP,37.29129010886,127.14838214123,181.8197,23.4000,0.0033,0.0013,-0.0007,0.575213789,0.437850468,245.200673613,0.6401,0.8201,1.0602,0.0013,0.0013,0.0011,0.5052,0.5141,0.0597,0f000055,0*c82d4eee\r\n#INSPVAXA,USB1,0,48.0,FINESTEERING,2089,274949.500,02000000,471d,15824;INS_SOLUTION_GOOD,INS_PSRSP,37.29129015687,127.14838223640,181.8108,23.4000,0.0038,0.0013,-0.0009,0.576341288,0.436502715,245.201339928,0.6372,0.8167,1.0547,0.0013,0.0013,0.0011,0.5051,0.5139,0.0598,0f000055,0*b2c63088\r\n#INSPVAXA,USB1,0,48.0,FINESTEERING,2089,274950.000,02000000,471d,15824;INS_SOLUTION_GOOD,INS_PSRSP,37.29129021208,127.14838233402,181.8018,23.4000,0.0037,0.0011,-0.0004,0.573177193,0.433662919,245.200620405,0.6372,0.8167,1.0547,0.0013,0.0013,0.0011,0.5051,0.5139,0.0598,0f000055,0*bb863ec0\r\n#INSPVAXA,USB1,0,47.5,FINESTEERING,2089,274950.500,02000000,471d,15824;INS_SOLUTION_GOOD,INS_PSRSP,37.29129025616,127.14838242498,181.7934,23.4000,0.0033,0.0011,0.0002,0.572555036,0.433594205,245.199426556,0.6342,0.8133,1.0493,0.0013,0.0013,0.0011,0.5050,0.5138,0.0597,0f000055,0*f11526f0\r\n#INSPVAXA,USB1,0,47.5,FINESTEERING,2089,274951.000,02000000,471d,15824;INS_SOLUTION_GOOD,INS_PSRSP,37.29129030551,127.14838251900,181.7853,23.4000,0.0025,0.0008,0.0013,0.572176766,0.431281506,245.199350122,0.6342,0.8133,1.0493,0.0013,0.0013,0.0011,0.5050,0.5138,0.0597,0f000055,0*d41cc7b1\r\n#INSPVAXA,USB1,0,47.5,FINESTEERING,2089,274951.500,02000000,471d,15824;INS_SOLUTION_GOOD,INS_PSRSP,37.29129034442,127.14838260933,181.7772,23.4000,0.0017,0.0014,0.0017,0.570144240,0.432300154,245.199383099,0.6314,0.8100,1.0440,0.0013,0.0013,0.0011,0.5049,0.5137,0.0596,0f000055,0*abb9ba6c\r\n#INSPVAXA,USB1,0,50.5,FINESTEERING,2089,274952.000,02000000,471d,15824;INS_SOLUTION_GOOD,INS_PSRSP,37.29129038640,127.14838270315,181.7694,23.4000,0.0016,0.0012,0.0022,0.571348600,0.430399864,245.195847291,0.6314,0.8100,1.0440,0.0013,0.0013,0.0011,0.5049,0.5137,0.0596,0f000055,0*e3c95238\r\n#INSPVAXA,USB1,0,50.0,FINESTEERING,2089,274952.500,02000000,471d,15824;INS_SOLUTION_GOOD,INS_PSRSP,37.29129043244,127.14838278253,181.7620,23.4000,0.0012,0.0004,0.0018,0.572029160,0.429673308,245.197267230,0.6285,0.8067,1.0388,0.0013,0.0013,0.0011,0.5047,0.5135,0.0594,0f000055,0*6f2b753a\r\n#INSPVAXA,USB1,0,50.0,FINESTEERING,2089,274953.000,02000000,471d,15824;INS_SOLUTION_GOOD,INS_PSRSP,37.29129048171,127.14838286368,181.7548,23.4000,0.0012,0.0008,0.0016,0.571374785,0.429419283,245.199544210,0.6285,0.8067,1.0388,0.0013,0.0013,0.0011,0.5047,0.5135,0.0594,0f000055,0*bd26dce1\r\n#INSPVAXA,USB1,0,49.5,FINESTEERING,2089,274953.500,02000000,471d,15824;INS_SOLUTION_GOOD,INS_PSRSP,37.29129052623,127.14838294740,181.7479,23.4000,0.0001,0.0011,0.0014,0.574183223,0.428084866,245.199190116,0.6257,0.8034,1.0336,0.0013,0.0013,0.0011,0.5047,0.5134,0.0592,0f000055,0*eab36f91\r\n#INSPVAXA,USB1,0,49.5,FINESTEERING,2089,274954.000,02000000,471d,15824;INS_SOLUTION_GOOD,INS_PSRSP,37.29129056824,127.14838303341,181.7410,23.4000,-0.0009,0.0007,0.0014,0.573188881,0.424856663,245.198405098,0.6257,0.8034,1.0336,0.0013,0.0013,0.0011,0.5047,0.5134,0.0592,0f000055,0*c1628286\r\n#INSPVAXA,USB1,0,44.5,FINESTEERING,2089,274954.500,02000000,471d,15824;INS_SOLUTION_GOOD,INS_PSRSP,37.29129061603,127.14838311267,181.7342,23.4000,-0.0014,0.0016,0.0014,0.572167091,0.425427466,245.196983276,0.6229,0.8002,1.0286,0.0013,0.0013,0.0011,0.5046,0.5133,0.0590,0f000055,0*abcc4a49\r\n#INSPVAXA,USB1,0,44.5,FINESTEERING,2089,274955.000,02000000,471d,15824;INS_SOLUTION_GOOD,INS_PSRSP,37.29129066072,127.14838319719,181.7279,23.4000,-0.0014,0.0023,0.0023,0.574657598,0.424857568,245.195420649,0.6229,0.8002,1.0286,0.0013,0.0013,0.0011,0.5046,0.5133,0.0590,0f000055,0*d57fed01\r\n#INSPVAXA,USB1,0,44.5,FINESTEERING,2089,274955.500,02000000,471d,15824;INS_SOLUTION_GOOD,INS_PSRSP,37.29129070969,127.14838327498,181.7215,23.4000,-0.0012,0.0018,0.0018,0.575229252,0.425372409,245.195942116,0.6201,0.7970,1.0236,0.0013,0.0013,0.0011,0.5045,0.5132,0.0587,0f000055,0*5832983e\r\n#INSPVAXA,USB1,0,50.0,FINESTEERING,2089,274956.000,02000000,471d,15824;INS_SOLUTION_GOOD,INS_PSRSP,37.29129075779,127.14838335627,181.7153,23.4000,-0.0004,0.0015,0.0015,0.579681238,0.425270111,245.198168548,0.6201,0.7970,1.0236,0.0013,0.0013,0.0011,0.5045,0.5132,0.0587,0f000055,0*81ba500b\r\n#INSPVAXA,USB1,0,50.0,FINESTEERING,2089,274956.500,02000000,471d,15824;INS_SOLUTION_GOOD,INS_PSRSP,37.29129080677,127.14838343176,181.7089,23.4000,0.0003,0.0004,0.0009,0.583026024,0.424223478,245.198710574,0.6174,0.7938,1.0187,0.0013,0.0013,0.0011,0.5044,0.5132,0.0585,0f000055,0*58f7b1b8\r\n#INSPVAXA,USB1,0,50.0,FINESTEERING,2089,274957.000,02000000,471d,15824;INS_SOLUTION_GOOD,INS_PSRSP,37.29129086261,127.14838350860,181.7025,23.4000,0.0022,0.0004,0.0009,0.584517852,0.425977961,245.199492067,0.6174,0.7938,1.0187,0.0013,0.0013,0.0011,0.5044,0.5132,0.0585,0f000055,0*9b834841\r\n#INSPVAXA,USB1,0,50.0,FINESTEERING,2089,274957.500,02000000,471d,15824;INS_SOLUTION_GOOD,INS_PSRSP,37.29129090862,127.14838358605,181.6968,23.4000,0.0029,0.0004,0.0011,0.583598016,0.426552938,245.198741013,0.6147,0.7907,1.0139,0.0013,0.0013,0.0011,0.5043,0.5131,0.0583,0f000055,0*91f8c5d3\r\n#INSPVAXA,USB1,0,52.0,FINESTEERING,2089,274958.000,02000000,471d,15824;INS_SOLUTION_GOOD,INS_PSRSP,37.29129096182,127.14838366575,181.6911,23.4000,0.0034,0.0012,0.0005,0.587557614,0.427026000,245.196843346,0.6147,0.7907,1.0139,0.0013,0.0013,0.0011,0.5043,0.5131,0.0583,0f000055,0*a25e153d\r\n#INSPVAXA,USB1,0,52.0,FINESTEERING,2089,274958.500,02000000,471d,15824;INS_SOLUTION_GOOD,INS_PSRSP,37.29129100175,127.14838374056,181.6849,23.4000,0.0033,0.0012,0.0009,0.584756996,0.426607543,245.200057711,0.6121,0.7876,1.0091,0.0013,0.0013,0.0011,0.5043,0.5130,0.0583,0f000055,0*66ea5405\r\n#INSPVAXA,USB1,0,52.0,FINESTEERING,2089,274959.000,02000000,471d,15824;INS_SOLUTION_GOOD,INS_PSRSP,37.29129104527,127.14838381896,181.6789,23.4000,0.0021,0.0014,0.0007,0.584527437,0.426853607,245.204834332,0.6121,0.7876,1.0091,0.0013,0.0013,0.0011,0.5043,0.5130,0.0583,0f000055,0*05c57504\r\n#INSPVAXA,USB1,0,52.0,FINESTEERING,2089,274959.500,02000000,471d,15824;INS_SOLUTION_GOOD,INS_PSRSP,37.29129108469,127.14838389047,181.6733,23.4000,0.0022,0.0019,0.0008,0.587402007,0.425657365,245.201828166,0.6095,0.7846,1.0044,0.0013,0.0013,0.0011,0.5042,0.5129,0.0585,0f000055,0*052a3b38\r\n#INSPVAXA,USB1,0,53.0,FINESTEERING,2089,274960.000,02000000,471d,15824;INS_SOLUTION_GOOD,INS_PSRSP,37.29129113139,127.14838396794,181.6679,23.4000,0.0033,0.0017,0.0011,0.589069004,0.423517039,245.198524386,0.6095,0.7846,1.0044,0.0013,0.0013,0.0011,0.5042,0.5129,0.0585,0f000055,0*fee6b9fb\r\n#INSPVAXA,USB1,0,47.0,FINESTEERING,2089,274960.500,02000000,471d,15824;INS_SOLUTION_GOOD,INS_PSRSP,37.29129117405,127.14838402539,181.6622,23.4000,0.0009,0.0006,0.0012,0.591017862,0.420907371,245.209720711,0.6072,0.7816,1.0000,0.0014,0.0014,0.0011,0.5041,0.5128,0.0598,0f000045,0*7f9afab6\r\n#INSPVAXA,USB1,0,47.0,FINESTEERING,2089,274961.000,02000000,471d,15824;INS_SOLUTION_GOOD,INS_PSRSP,37.29129121933,127.14838408427,181.6569,23.4000,0.0013,-0.0004,0.0029,0.583607279,0.422224912,245.201730981,0.6072,0.7816,1.0000,0.0014,0.0014,0.0011,0.5041,0.5128,0.0598,0f000045,0*e87f76df\r\n#INSPVAXA,USB1,0,47.0,FINESTEERING,2089,274961.500,02000000,471d,15824;INS_SOLUTION_GOOD,INS_PSRSP,37.29129127982,127.14838417720,181.6536,23.4000,0.0032,0.0002,0.0022,0.589088944,0.421521547,245.198660735,0.6055,0.7791,0.9960,0.0094,0.0094,0.0088,0.5042,0.5130,0.0613,0f000051,0*3d9a419b\r\n#INSPVAXA,USB1,0,49.0,FINESTEERING,2089,274962.000,02000000,471d,15824;INS_SOLUTION_GOOD,INS_PSRSP,37.29129134550,127.14838427298,181.6506,23.4000,0.0022,0.0011,0.0029,0.591327857,0.423201142,245.198914785,0.6055,0.7791,0.9960,0.0094,0.0094,0.0088,0.5042,0.5130,0.0613,0f000051,0*01a6c642\r\n#INSPVAXA,USB1,0,49.0,FINESTEERING,2089,274962.500,02000000,471d,15824;INS_SOLUTION_GOOD,INS_PSRSP,37.29129138241,127.14838435910,181.6456,23.4000,0.0014,0.0013,0.0028,0.593286002,0.425262248,245.187899073,0.6028,0.7759,0.9914,0.0014,0.0014,0.0011,0.5039,0.5127,0.0631,0f000055,0*6c98b2f1\r\n#INSPVAXA,USB1,0,50.5,FINESTEERING,2089,274963.000,02000000,471d,15824;INS_SOLUTION_GOOD,INS_PSRSP,37.29129141750,127.14838444748,181.6409,23.4000,0.0015,0.0009,0.0026,0.596301579,0.427685435,245.181860150,0.6028,0.7759,0.9914,0.0014,0.0014,0.0011,0.5039,0.5127,0.0631,0f000055,0*508c7444\r\n#INSPVAXA,USB1,0,50.5,FINESTEERING,2089,274963.500,02000000,471d,15824;INS_SOLUTION_GOOD,INS_PSRSP,37.29129145846,127.14838452836,181.6361,23.4000,0.0016,0.0011,0.0009,0.594301534,0.432635960,245.182713950,0.6004,0.7730,0.9871,0.0014,0.0014,0.0011,0.5037,0.5126,0.0649,0f000055,0*f3a5a760\r\n#INSPVAXA,USB1,0,51.5,FINESTEERING,2089,274964.000,02000000,471d,15824;INS_SOLUTION_GOOD,INS_PSRSP,37.29129150712,127.14838461507,181.6312,23.4000,0.0030,0.0011,-0.0007,0.595109644,0.435637175,245.181773224,0.6004,0.7730,0.9871,0.0014,0.0014,0.0011,0.5037,0.5126,0.0649,0f000055,0*4dcac95b\r\n#INSPVAXA,USB1,0,50.0,FINESTEERING,2089,274964.500,02000000,471d,15824;INS_SOLUTION_GOOD,INS_PSRSP,37.29129154600,127.14838469136,181.6273,23.4000,0.0022,0.0001,-0.0009,0.603360806,0.432839407,245.172365629,0.5981,0.7702,0.9828,0.0014,0.0014,0.0011,0.5037,0.5125,0.0663,0f000055,0*3f5a10c0\r\n#INSPVAXA,USB1,0,50.0,FINESTEERING,2089,274965.000,02000000,471d,15824;INS_SOLUTION_GOOD,INS_PSRSP,37.29129158713,127.14838476659,181.6232,23.4000,0.0011,0.0001,-0.0012,0.596555358,0.428746150,245.163728698,0.5981,0.7702,0.9828,0.0014,0.0014,0.0011,0.5037,0.5125,0.0663,0f000055,0*d82bb08b\r\n#INSPVAXA,USB1,0,50.0,FINESTEERING,2089,274965.500,02000000,471d,15824;INS_SOLUTION_GOOD,INS_PSRSP,37.29129162132,127.14838485034,181.6195,23.4000,-0.0006,0.0003,-0.0008,0.596864595,0.431764594,245.151905668,0.5958,0.7674,0.9786,0.0014,0.0014,0.0011,0.5036,0.5124,0.0674,0f000055,0*1ec93ee4\r\n#INSPVAXA,USB1,0,50.5,FINESTEERING,2089,274966.000,02000000,471d,15824;INS_SOLUTION_GOOD,INS_PSRSP,37.29129165663,127.14838493529,181.6158,23.4000,-0.0002,-0.0003,0.0011,0.595541957,0.432552534,245.143660464,0.5958,0.7674,0.9786,0.0014,0.0014,0.0011,0.5036,0.5124,0.0674,0f000055,0*6e129fc1\r\n#INSPVAXA,USB1,0,46.5,FINESTEERING,2089,274966.500,02000000,471d,15824;INS_SOLUTION_GOOD,INS_PSRSP,37.29129169307,127.14838500599,181.6119,23.4000,-0.0009,-0.0014,0.0009,0.596677381,0.430178197,245.136787932,0.5936,0.7646,0.9745,0.0014,0.0014,0.0011,0.5035,0.5123,0.0684,0f000055,0*6fe0c265\r\n#INSPVAXA,USB1,0,46.5,FINESTEERING,2089,274967.000,02000000,471d,15824;INS_SOLUTION_GOOD,INS_PSRSP,37.29129173334,127.14838507823,181.6082,23.4000,-0.0006,-0.0003,-0.0007,0.592977234,0.431347828,245.127161786,0.5936,0.7646,0.9745,0.0014,0.0014,0.0011,0.5035,0.5123,0.0684,0f000055,0*873c14c7\r\n#INSPVAXA,USB1,0,46.5,FINESTEERING,2089,274967.500,02000000,471d,15824;INS_SOLUTION_GOOD,INS_PSRSP,37.29129178115,127.14838516128,181.6061,23.4000,0.0031,-0.0027,0.0015,0.591180173,0.435814263,245.120136007,0.5914,0.7619,0.9705,0.0014,0.0014,0.0011,0.5034,0.5122,0.0691,0f000055,0*7383a626\r\n#INSPVAXA,USB1,0,49.5,FINESTEERING,2089,274968.000,02000000,471d,15824;INS_SOLUTION_GOOD,INS_PSRSP,37.29129183174,127.14838524440,181.6043,23.4000,0.0025,0.0013,0.0038,0.595515669,0.441370278,245.129863964,0.5914,0.7619,0.9705,0.0014,0.0014,0.0011,0.5034,0.5122,0.0691,0f000055,0*0daebb7a\r\n#INSPVAXA,USB1,0,47.5,FINESTEERING,2089,274968.500,02000000,471d,15824;INS_SOLUTION_GOOD,INS_PSRSP,37.29129185905,127.14838530634,181.5996,23.4000,0.0018,0.0005,0.0024,0.595471635,0.437472405,245.134128753,0.5893,0.7593,0.9665,0.0014,0.0014,0.0011,0.5032,0.5120,0.0695,0f000055,0*8aa14461\r\n#INSPVAXA,USB1,0,47.5,FINESTEERING,2089,274969.000,02000000,471d,15824;INS_SOLUTION_GOOD,INS_PSRSP,37.29129189262,127.14838536968,181.5949,23.4000,0.0017,-0.0008,0.0011,0.597333777,0.435726572,245.133708870,0.5893,0.7593,0.9665,0.0014,0.0014,0.0011,0.5032,0.5120,0.0695,0f000055,0*2b473198\r\n#INSPVAXA,USB1,0,47.5,FINESTEERING,2089,274969.500,02000000,471d,15824;INS_SOLUTION_GOOD,INS_PSRSP,37.29129193110,127.14838544063,181.5916,23.4000,0.0021,-0.0012,0.0014,0.596034182,0.434848319,245.130924723,0.5873,0.7567,0.9627,0.0014,0.0014,0.0011,0.5031,0.5120,0.0696,0f000055,0*fadaa671\r\n#INSPVAXA,USB1,0,47.5,FINESTEERING,2089,274970.000,02000000,471d,15824;INS_SOLUTION_GOOD,INS_PSRSP,37.29129197844,127.14838550745,181.5886,23.4000,0.0041,-0.0014,0.0020,0.595546179,0.434121459,245.124984065,0.5873,0.7567,0.9627,0.0014,0.0014,0.0011,0.5031,0.5120,0.0696,0f000055,0*6980795b\r\n#INSPVAXA,USB1,0,45.5,FINESTEERING,2089,274970.500,02000000,471d,15824;INS_SOLUTION_GOOD,INS_PSRSP,37.29129201031,127.14838557276,181.5851,23.4000,0.0039,-0.0014,0.0019,0.597356777,0.433113363,245.126670277,0.5853,0.7541,0.9589,0.0014,0.0014,0.0011,0.5030,0.5119,0.0696,0f000055,0*f2e18748\r\n#INSPVAXA,USB1,0,45.5,FINESTEERING,2089,274971.000,02000000,471d,15824;INS_SOLUTION_GOOD,INS_PSRSP,37.29129205180,127.14838563798,181.5822,23.4000,0.0044,-0.0012,0.0020,0.591930037,0.430882356,245.128692169,0.5853,0.7541,0.9589,0.0014,0.0014,0.0011,0.5030,0.5119,0.0696,0f000055,0*57eebc53\r\n#INSPVAXA,USB1,0,45.5,FINESTEERING,2089,274971.500,02000000,471d,15824;INS_SOLUTION_GOOD,INS_PSRSP,37.29129208007,127.14838570576,181.5792,23.4000,0.0032,-0.0015,0.0026,0.591416897,0.429504649,245.118719014,0.5833,0.7516,0.9551,0.0013,0.0013,0.0011,0.5029,0.5118,0.0694,0f000055,0*a9b9e7dc\r\n#INSPVAXA,USB1,0,46.0,FINESTEERING,2089,274972.000,02000000,471d,15824;INS_SOLUTION_GOOD,INS_PSRSP,37.29129211114,127.14838577057,181.5766,23.4000,0.0030,-0.0015,0.0027,0.591399554,0.429092210,245.111731050,0.5833,0.7516,0.9551,0.0013,0.0013,0.0011,0.5029,0.5118,0.0694,0f000055,0*9e2f22a3\r\n#INSPVAXA,USB1,0,46.0,FINESTEERING,2089,274972.500,02000000,471d,15824;INS_SOLUTION_GOOD,INS_PSRSP,37.29129214411,127.14838583379,181.5730,23.4000,0.0040,-0.0010,0.0017,0.593530073,0.432268075,245.109171805,0.5814,0.7492,0.9515,0.0013,0.0013,0.0011,0.5028,0.5117,0.0692,0f000055,0*c98e6d62\r\n#INSPVAXA,USB1,0,46.0,FINESTEERING,2089,274973.000,02000000,471d,15824;INS_SOLUTION_GOOD,INS_PSRSP,37.29129218492,127.14838589703,181.5697,23.4000,0.0036,-0.0014,0.0018,0.597236592,0.434427742,245.111916475,0.5814,0.7492,0.9515,0.0013,0.0013,0.0011,0.5028,0.5117,0.0692,0f000055,0*3a1cba8f\r\n#INSPVAXA,USB1,0,46.0,FINESTEERING,2089,274973.500,02000000,471d,15824;INS_SOLUTION_GOOD,INS_PSRSP,37.29129220943,127.14838595196,181.5679,23.4000,0.0037,-0.0022,0.0022,0.590920237,0.435249318,245.120230153,0.5795,0.7467,0.9479,0.0013,0.0013,0.0011,0.5027,0.5116,0.0690,0f000055,0*9e9cb60a\r\n#INSPVAXA,USB1,0,50.0,FINESTEERING,2089,274974.000,02000000,471d,15824;INS_SOLUTION_GOOD,INS_PSRSP,37.29129223622,127.14838600066,181.5662,23.4000,0.0024,-0.0031,0.0019,0.592046212,0.434673577,245.128673665,0.5795,0.7467,0.9479,0.0013,0.0013,0.0011,0.5027,0.5116,0.0690,0f000055,0*8773c9cf\r\n#INSPVAXA,USB1,0,48.0,FINESTEERING,2089,274974.500,02000000,471d,15824;INS_SOLUTION_GOOD,INS_PSRSP,37.29129225936,127.14838606194,181.5629,23.4000,0.0018,-0.0033,0.0021,0.588427984,0.436117345,245.120879814,0.5777,0.7444,0.9444,0.0013,0.0013,0.0011,0.5024,0.5115,0.0688,0f000055,0*a6d78863\r\n#INSPVAXA,USB1,0,48.0,FINESTEERING,2089,274975.000,02000000,471d,15824;INS_SOLUTION_GOOD,INS_PSRSP,37.29129228451,127.14838611946,181.5594,23.4000,0.0016,-0.0024,0.0006,0.589014138,0.438636504,245.113459226,0.5777,0.7444,0.9444,0.0013,0.0013,0.0011,0.5024,0.5115,0.0688,0f000055,0*e67a0118\r\n#INSPVAXA,USB1,0,48.0,FINESTEERING,2089,274975.500,02000000,471d,15824;INS_SOLUTION_GOOD,INS_PSRSP,37.29129231232,127.14838617825,181.5566,23.4000,0.0023,-0.0020,0.0007,0.583384275,0.439887421,245.110738283,0.5759,0.7421,0.9409,0.0013,0.0013,0.0011,0.5024,0.5115,0.0685,0f000055,0*dd1d55ce\r\n#INSPVAXA,USB1,0,50.0,FINESTEERING,2089,274976.000,02000000,471d,15824;INS_SOLUTION_GOOD,INS_PSRSP,37.29129234327,127.14838623434,181.5543,23.4000,0.0016,-0.0021,0.0013,0.584731257,0.441970314,245.107275137,0.5759,0.7421,0.9409,0.0013,0.0013,0.0011,0.5024,0.5115,0.0685,0f000055,0*fc31a58d\r\n#INSPVAXA,USB1,0,46.0,FINESTEERING,2089,274976.500,02000000,471d,15824;INS_SOLUTION_GOOD,INS_PSRSP,37.29129236683,127.14838629592,181.5517,23.4000,0.0012,-0.0021,0.0021,0.586209347,0.445368862,245.103009782,0.5742,0.7400,0.9376,0.0013,0.0013,0.0011,0.5022,0.5113,0.0684,0f000055,0*2f762464\r\n#INSPVAXA,USB1,0,46.0,FINESTEERING,2089,274977.000,02000000,471d,15824;INS_SOLUTION_GOOD,INS_PSRSP,37.29129238644,127.14838635054,181.5496,23.4000,-0.0006,-0.0025,0.0026,0.582043222,0.447512293,245.101489371,0.5742,0.7400,0.9376,0.0013,0.0013,0.0011,0.5022,0.5113,0.0684,0f000055,0*f6c031e0\r\n#INSPVAXA,USB1,0,46.0,FINESTEERING,2089,274977.500,02008000,471d,15824;INS_SOLUTION_GOOD,INS_PSRSP,37.29129241405,127.14838640703,181.5464,23.4000,0.0008,-0.0010,0.0018,0.579730709,0.452676443,245.094649730,0.5726,0.7377,0.9343,0.0013,0.0013,0.0011,0.5021,0.5112,0.0682,0f000055,0*bae2da46\r\n#INSPVAXA,USB1,0,49.5,FINESTEERING,2089,274978.000,02008000,471d,15824;INS_SOLUTION_GOOD,INS_PSRSP,37.29129244543,127.14838646623,181.5433,23.4000,0.0012,0.0003,0.0008,0.583220842,0.454096324,245.089395626,0.5726,0.7377,0.9343,0.0013,0.0013,0.0011,0.5021,0.5112,0.0682,0f000055,0*a6b5b51c\r\n#INSPVAXA,USB1,0,46.0,FINESTEERING,2089,274978.500,02008000,471d,15824;INS_SOLUTION_GOOD,INS_PSRSP,37.29129246784,127.14838651613,181.5406,23.4000,0.0013,0.0012,0.0008,0.583568601,0.454470356,245.089692497,0.5708,0.7355,0.9309,0.0013,0.0013,0.0011,0.5020,0.5111,0.0679,0f000055,0*58c15f15\r\n#INSPVAXA,USB1,0,46.0,FINESTEERING,2089,274979.000,02008000,471d,15824;INS_SOLUTION_GOOD,INS_PSRSP,37.29129249649,127.14838657330,181.5382,23.4000,0.0024,0.0022,0.0007,0.583596243,0.454905157,245.090634601,0.5708,0.7355,0.9309,0.0013,0.0013,0.0011,0.5020,0.5111,0.0679,0f000055,0*1fc0baeb\r\n#INSPVAXA,USB1,0,46.0,FINESTEERING,2089,274979.500,02008000,471d,15824;INS_SOLUTION_GOOD,INS_PSRSP,37.29129251917,127.14838662144,181.5359,23.4000,0.0020,0.0016,0.0010,0.586578002,0.452597521,245.083972280,0.5691,0.7332,0.9276,0.0013,0.0013,0.0011,0.5019,0.5111,0.0676,0f000055,0*031b83c9\r\n#INSPVAXA,USB1,0,48.0,FINESTEERING,2089,274980.000,02008000,471d,15824;INS_SOLUTION_GOOD,INS_PSRSP,37.29129254945,127.14838667155,181.5338,23.4000,0.0036,0.0009,0.0005,0.588660941,0.450809595,245.079452294,0.5691,0.7332,0.9276,0.0013,0.0013,0.0011,0.5019,0.5111,0.0676,0f000055,0*027169f5\r\n#INSPVAXA,USB1,0,45.5,FINESTEERING,2089,274980.500,02008000,471d,15824;INS_SOLUTION_GOOD,INS_PSRSP,37.29129257137,127.14838671360,181.5307,23.4000,0.0031,0.0007,0.0001,0.588220567,0.451946553,245.078601977,0.5673,0.7310,0.9243,0.0013,0.0013,0.0011,0.5018,0.5110,0.0678,0f000045,0*0b1bcae4\r\n#INSPVAXA,USB1,0,45.5,FINESTEERING,2089,274981.000,02008000,471d,15824;INS_SOLUTION_GOOD,INS_PSRSP,37.29129259982,127.14838675511,181.5278,23.4000,0.0034,0.0001,0.0002,0.589879061,0.455338936,245.078019282,0.5673,0.7310,0.9243,0.0013,0.0013,0.0011,0.5018,0.5110,0.0678,0f000045,0*d93e2d27\r\n#INSPVAXA,USB1,0,45.5,FINESTEERING,2089,274981.500,02008000,471d,15824;INS_SOLUTION_GOOD,INS_PSRSP,37.29129263099,127.14838681784,181.5275,23.4000,0.0018,-0.0004,0.0010,0.587573769,0.457809446,245.070973222,0.5659,0.7291,0.9213,0.0013,0.0013,0.0011,0.5017,0.5109,0.0676,0f000055,0*f255b369\r\n#INSPVAXA,USB1,0,48.0,FINESTEERING,2089,274982.000,02000000,471d,15824;INS_SOLUTION_GOOD,INS_PSRSP,37.29129266154,127.14838688357,181.5277,23.4000,0.0002,0.0002,0.0022,0.587590681,0.459988173,245.065903820,0.5659,0.7291,0.9213,0.0013,0.0013,0.0011,0.5017,0.5109,0.0676,0f000055,0*a8f1c6c9\r\n#INSPVAXA,USB1,0,45.5,FINESTEERING,2089,274982.500,02000000,471d,15824;INS_SOLUTION_GOOD,INS_PSRSP,37.29129271863,127.14838691961,181.5198,23.4000,0.0008,0.0006,0.0023,0.593617397,0.460236893,245.059822692,0.5639,0.7278,0.9182,0.0013,0.0013,0.0011,0.5016,0.5107,0.0675,0f000055,0*2afab1e0\r\n#INSPVAXA,USB1,0,45.5,FINESTEERING,2089,274983.000,02000000,471d,15824;INS_SOLUTION_GOOD,INS_PSRSP,37.29129278279,127.14838695677,181.5117,23.4000,0.0022,0.0009,0.0013,0.597323864,0.457896470,245.051677508,0.5639,0.7278,0.9182,0.0013,0.0013,0.0011,0.5016,0.5107,0.0675,0f000055,0*9cce4e5d\r\n#INSPVAXA,USB1,0,45.5,FINESTEERING,2089,274983.500,02000000,471d,15824;INS_SOLUTION_GOOD,INS_PSRSP,37.29129283560,127.14838699355,181.5029,23.4000,0.0025,0.0008,0.0007,0.594795177,0.456732941,245.048392236,0.5620,0.7256,0.9149,0.0013,0.0013,0.0011,0.5015,0.5106,0.0673,0f000055,0*32fb5065\r\n#INSPVAXA,USB1,0,50.0,FINESTEERING,2089,274984.000,02000000,471d,15824;INS_SOLUTION_GOOD,INS_PSRSP,37.29129289489,127.14838703333,181.4939,23.4000,0.0020,0.0010,-0.0000,0.589856266,0.455434649,245.044401998,0.5620,0.7256,0.9149,0.0013,0.0013,0.0011,0.5015,0.5106,0.0673,0f000055,0*a69ab41d\r\n#INSPVAXA,USB1,0,46.0,FINESTEERING,2089,274984.500,02000000,471d,15824;INS_SOLUTION_GOOD,INS_PSRSP,37.29129295510,127.14838708601,181.4852,23.4000,0.0033,0.0005,0.0001,0.585743432,0.456583423,245.043163281,0.5601,0.7235,0.9116,0.0013,0.0013,0.0011,0.5014,0.5106,0.0670,0f000055,0*b267cfbf\r\n#INSPVAXA,USB1,0,46.0,FINESTEERING,2089,274985.000,02000000,471d,15824;INS_SOLUTION_GOOD,INS_PSRSP,37.29129302384,127.14838714153,181.4764,23.4000,0.0038,0.0007,0.0001,0.583712648,0.457384559,245.042978117,0.5601,0.7235,0.9116,0.0013,0.0013,0.0011,0.5014,0.5106,0.0670,0f000055,0*ce3c1a70\r\n#INSPVAXA,USB1,0,46.0,FINESTEERING,2089,274985.500,02000000,471d,15824;INS_SOLUTION_GOOD,INS_PSRSP,37.29129307741,127.14838717759,181.4683,23.4000,0.0044,0.0006,0.0002,0.583864383,0.456689574,245.042936428,0.5584,0.7215,0.9083,0.0013,0.0013,0.0011,0.5014,0.5105,0.0665,0f000055,0*9ac9e3ac\r\n"
  out "GPS Data":T1={"Latitude"={"Valid?"=TRUE, "Latitude (Deg)"=37.37123095061}, "Longitude"={"Valid?"=TRUE, "Longitude (Deg)"=126.72256864175}, "Height"={"Valid?"=TRUE, "Height (m)"=9.9059}, "Undulation"={"Valid?"=TRUE, "Undulation(m)"=22.3}, "North Vel"={"Valid?"=TRUE, "North Vel (m/s)"=-0.0013}, "East Vel"={"Valid?"=TRUE, "East Vel (m/s)"=-0.002}, "Up Vel"={"Valid?"=TRUE, "Up Vel (m/s)"=0.0004}, "Roll"={"Valid?"=TRUE, "Roll (degrees)"=-0.425709275}, "Pitch"={"Valid?"=TRUE, "Pitch (degrees)"=-0.898393069}, "Azimuth"={"Valid?"=TRUE, "Azimuth (degrees)"=98.594488749}, "Lat deviation"={"Valid?"=TRUE, "Lat deviation (m)"=0.4755}, "Long deviation"={"Valid?"=TRUE, "Long deviation (m)"=0.4754}, "Height deviation"={"Valid?"=TRUE, "Height deviation (m)"=0.9034}, "North vel deviation"={"Valid?"=TRUE, "North vel deviation (m/s)"=0.0181}, "East vel deviation"={"Valid?"=TRUE, "East vel deviation (m/s)"=0.018}, "Up vel deviation"={"Valid?"=TRUE, "Up vel deviation (m/s)"=0.0196}, "Roll deviation"={"Valid?"=TRUE, "Roll deviation (degrees)"=0.0309}, "Pitch deviation"={"Valid?"=TRUE, "Pitch deviation (degrees)"=0.0311}, "Azimuth deviation"={"Valid?"=TRUE, "Azimuth deviation (degrees)"=0.1368}, "Ext sol status"={"Valid?"=TRUE, "Ext sol status"=0.0}}
  out "Heading":dbl=98.684623718
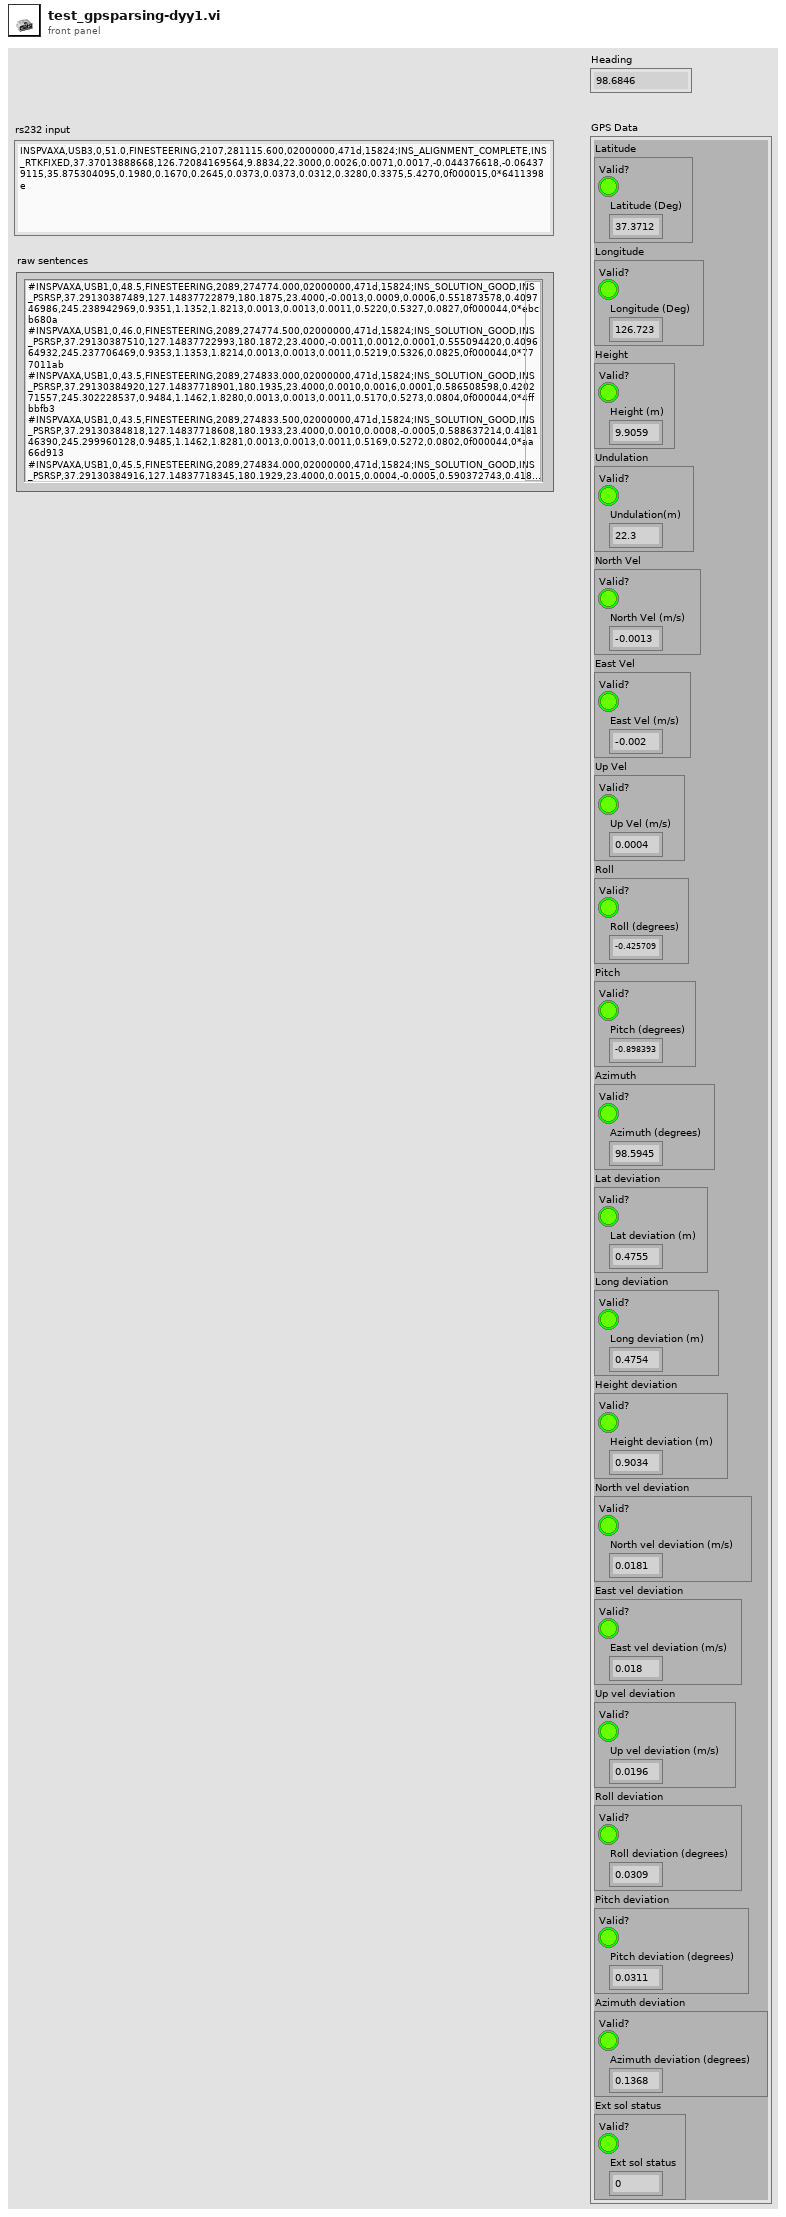
[diagram p1: front panel]
types:
  T1 = cluster{"Latitude":cluster{"Valid?":bool, "Latitude (Deg)":dbl}, "Longitude":cluster{"Valid?":bool, "Longitude (Deg)":dbl}, "Height":cluster{"Valid?":bool, "Height (m)":dbl}, "Undulation":cluster{"Valid?":bool, "Undulation(m)":dbl}, "North Vel":cluster{"Valid?":bool, "North Vel (m/s)":dbl}, "East Vel":cluster{"Valid?":bool, "East Vel (m/s)":dbl}, "Up Vel":cluster{"Valid?":bool, "Up Vel (m/s)":dbl}, "Roll":cluster{"Valid?":bool, "Roll (degrees)":dbl}, "Pitch":cluster{"Valid?":bool, "Pitch (degrees)":dbl}, "Azimuth":cluster{"Valid?":bool, "Azimuth (degrees)":dbl}, "Lat deviation":cluster{"Valid?":bool, "Lat deviation (m)":dbl}, "Long deviation":cluster{"Valid?":bool, "Long deviation (m)":dbl}, "Height deviation":cluster{"Valid?":bool, "Height deviation (m)":dbl}, "North vel deviation":cluster{"Valid?":bool, "North vel deviation (m/s)":dbl}, "East vel deviation":cluster{"Valid?":bool, "East vel deviation (m/s)":dbl}, "Up vel deviation":cluster{"Valid?":bool, "Up vel deviation (m/s)":dbl}, "Roll deviation":cluster{"Valid?":bool, "Roll deviation (degrees)":dbl}, "Pitch deviation":cluster{"Valid?":bool, "Pitch deviation (degrees)":dbl}, "Azimuth deviation":cluster{"Valid?":bool, "Azimuth deviation (degrees)":dbl}, "Ext sol status":cluster{"Valid?":bool, "Ext sol status":dbl}}
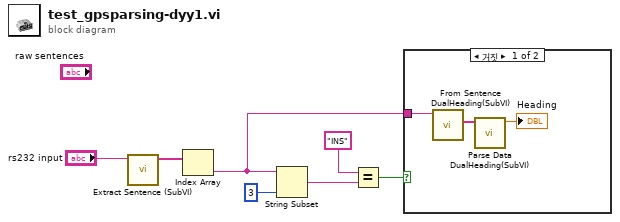
[diagram p0: block diagram]
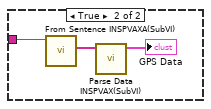
[diagram p2: hidden frame]
diagram:
  n1 = call "Extract Sentence (SubVI).vi"("raw sentences"="rs232 input") -> ("extract sentences"=w7:string[])  [unwired: 10 in]
  n2 = Index Array(array=w7) -> (element=w3:string)  [unwired: 1 in]
  n3 = String Subset(string=w3, length (rest)=3 ("길이(나머지)")) -> (substring=w5:string)  [unwired: 1 in]
  n4 = Equal?(x="INS", y=w5) -> (x = y?=w2:bool)
  n5 = case shown="거짓" w2 {
    tunnel: w3 -> [w8 w13]
    frame False {
      n6 = call "From Sentence DualHeading(SubVI).vi"("Extract Sentence"=w8) -> ("Parse Data Array"=w10:string[])  [unwired: 9 in, 1 out]
      n7 = call "Parse Data DualHeading(SubVI).vi"("Parse Data Array"=w10) -> ("Heading"=→"Heading":dbl)  [unwired: 10 in]
    }
    frame True {
      n8 = call "From Sentence INSPVAXA(SubVI).vi"("Extract Sentence"=w13) -> ("Parse Data Array"=w12:string[])  [unwired: 9 in, 1 out]
      n9 = call "Parse Data INSPVAX(SubVI).vi"("Parse Data Array"=w12) -> ("output cluster"=→"GPS Data":T1)  [unwired: 10 in]
    }
  }
